vi "dI-dV(V) at various H_MFLI_MF-MD_K3636B(channelB)_measureX_PK_V4.0_withaveraging.vi"() -> ()   [LabVIEW 2016]
uses:
  <instrlib>/Zurich Instruments LabOne/Public/Data/ziTypeDemodSampleSingle.ctl
  <instrlib>/Keithley 2600 Series/Public/Configure/Source/Configure Source (Limit).vi
  <instrlib>/Keithley 2600 Series/Public/Configure/Source/Configure Source (Range).vi
  <instrlib>/Zurich Instruments LabOne/Public/Configure/ziSetValueDouble.vi
  <instrlib>/Zurich Instruments LabOne/Public/Configure/ziGetValueDemodSampleEx.vi
  <instrlib>/Zurich Instruments LabOne/Zurich Instruments LabOne.lvlib
  <instrlib>/Keithley 2600 Series/Keithley 2600 Series.lvlib
panel:
  in  "MFLI autophase":bool
  in  "MFLI autorange":bool
  in  "MFLI averaging":i32=20
  in  "Resistance used for DC (ohm)":dbl=20000000.0 format="%#_13g"
  in  "DC Current Limit (A)":dbl=0.001 format="%#_13g"
  in  "Keithley 2636B (channelB)":refnum<visa-resource-name>="GPIB0::26::INSTR"
  in  "Field ramp rate (T/min)":string="0.05"
  in  "Step 2":dbl[](array[numeric])=[0.01] min=-3000.0 max=3000.0 format="%.1e"
  in  "To 2":dbl[](array[numeric])=[0.3] min=-3000.0 max=3000.0 format="%.1e"
  in  "From 2":dbl[](array[numeric])=[0.0] min=-3000.0 max=3000.0 format="%.1e"
  in  "Magnet IP Address":string="169.254.13.196"
  in  "Magnetic field stabilization time (s)":dbl=10.0 format="%#_13g"
  out "Magnetic Field (T)":dbl=-3.778e-06 format="%#_13g"
  in  "DC Voltage averaging":dbl=20.0 format="%#_13g"
  out "Demod Sample Out 2":T1={"Timestamps (ticks)"=128778643837950, "X (Vrms)"=2.3166004932731997e-10, "Y (Vrms)"=-1.6838016027024e-10, "Osc Phase (deg)"=2.502497907836938, "Freq (Hz)"=137.91900016713043, "DIO"=0, "AuxIn0 (V)"=-1.6014270555751864, "AuxIn1 (V)"=0.0003336581285111606, "Trigger"=768}
  out "Demod Sample Out":T1={"Timestamps (ticks)"=128778342710270, "X (Vrms)"=1.6896364938522627e-05, "Y (Vrms)"=-1.248107801044493e-05, "Osc Phase (deg)"=1.3353302758544507, "Freq (Hz)"=137.91900016713043, "DIO"=0, "AuxIn0 (V)"=-1.6014270555751864, "AuxIn1 (V)"=-0.0013346325140446424, "Trigger"=0}
  out "Vset (V)":dbl=-1.5999999999999879
  in  "stop":bool
  out "Time(s)":dbl=17571.544
  in  "Delay (s)":dbl=4.0
  out "dI/dV (S)":dbl=1.3582224457345251e-05
  out "dV (V)":dbl=1.6935759280791425e-05
  out "dI (A)":dbl=2.300252839072771e-10
  in  "MFLI Address":string="DEV4496"
  out "DC Voltage (V)":dbl=0.0024181997905000007
  in  "Folder":path=path "D:/Pranava/Data/Pt-Co-Ta/25-05-2021"
  out "dI/dV vs DC Bias (V)":cluster{dbl, "Field Reading":dbl}[](graph)=[{-0.001627013885, "Field Reading"=1.6344764120468297e-05}, {-0.001619012798, "Field Reading"=1.3998765196903891e-05}, {-0.0016148306399999999, "Field Reading"=1.3700556199628512e-05}, {-0.0016116390899999999, "Field Reading"=1.3871656998400836e-05}, {-0.0016093190579999999, "Field Reading"=1.3890284519929273e-05}, {-0.0016034726325000002, "Field Reading"=1.3832673860262865e-05}, {-0.0016014351899999997, "Field Reading"=1.3751553995812428e-05}, {-0.0015951204535000004, "Field Reading"=1.3732003453418088e-05}, {-0.001597877244, "Field Reading"=1.3898216235721011e-05}, {-0.0015940734674999998, "Field Reading"=1.3997320460561689e-05}, {-0.0015882617540000001, "Field Reading"=1.3508618550371427e-05}, {-0.0015828277630000002, "Field Reading"=1.367402259462331e-05}, {-0.0015791635179999998, "Field Reading"=1.3527207584083079e-05}, {-0.0015766756889999997, "Field Reading"=1.3882099502793414e-05}, {-0.00157194422, "Field Reading"=1.3768418031370217e-05}, {-0.0015670328779999998, "Field Reading"=1.364782208277766e-05}, {-0.0015644425175, "Field Reading"=1.3804633828353077e-05}, {-0.001564032793, "Field Reading"=1.3888199858922033e-05}, {-0.001557341777, "Field Reading"=1.3614302852212391e-05}, {-0.001552385615, "Field Reading"=1.3810158703062188e-05}, {-0.0015469061994999999, "Field Reading"=1.3764713120794011e-05}, {-0.001546229423, "Field Reading"=1.369552113795401e-05}, {-0.0015404441190000001, "Field Reading"=1.3693812113712007e-05}, {-0.0015395130355, "Field Reading"=1.3781883943418925e-05}, {-0.0015314868149999999, "Field Reading"=1.3770965025421842e-05}, {-0.0015304288265, "Field Reading"=1.3798857346413868e-05}, {-0.001527220823, "Field Reading"=1.3715545304114617e-05}, {-0.0015249214555, "Field Reading"=1.3691708736082112e-05}, {-0.0015218840245, "Field Reading"=1.3708493049006325e-05}, {-0.001520791987, "Field Reading"=1.3817916720703356e-05}, {-0.0015147427645, "Field Reading"=1.3894961593511675e-05}, {-0.001517215882, "Field Reading"=1.3590033991382936e-05}, {-0.0015114531689999998, "Field Reading"=1.3756144247138902e-05}, {-0.0015093745215, "Field Reading"=1.377966465179012e-05}, {-0.001500627891, "Field Reading"=1.3951323244665344e-05}, {-0.0015025901485, "Field Reading"=1.3667118977084549e-05}, {-0.0014961112455, "Field Reading"=1.3773922587587749e-05}, {-0.001492517136, "Field Reading"=1.3885930772190326e-05}, {-0.0014830039544999998, "Field Reading"=1.401422781639763e-05}, {-0.0014816401655, "Field Reading"=1.397897771474187e-05}, {-0.00147841159, "Field Reading"=1.379012752602543e-05}, {-0.0014741321355, "Field Reading"=1.3677898377939856e-05}, {-0.0014710702515, "Field Reading"=1.3843469527200954e-05}, {-0.0014655690059999999, "Field Reading"=1.3916776180729468e-05}, {-0.0014595854975000002, "Field Reading"=1.3757666149806165e-05}, {-0.0014580961389999997, "Field Reading"=1.3700038667069656e-05}, {-0.0014554962550000002, "Field Reading"=1.3953242012805934e-05}, {-0.0014536663915, "Field Reading"=1.3900636198435842e-05}, {-0.0014442646640000002, "Field Reading"=1.3742972292234844e-05}, {-0.001445856694, "Field Reading"=1.3937226017817598e-05}, {-0.0014406852145, "Field Reading"=1.3857514292073597e-05}, {-0.0014354871654999998, "Field Reading"=1.4045929404858086e-05}, {-0.001434501668, "Field Reading"=1.4042163913670806e-05}, {-0.0014285742130000002, "Field Reading"=1.3914255657909023e-05}, {-0.001420600119, "Field Reading"=1.3960330416901324e-05}, {-0.00142239087, "Field Reading"=1.387496710959369e-05}, {-0.001420244116, "Field Reading"=1.3967109128526288e-05}, {-0.0014127562885, "Field Reading"=1.3875867237048908e-05}, {-0.001408771663, "Field Reading"=1.371589748742955e-05}, {-0.001407767006, "Field Reading"=1.3711464298673438e-05}, {-0.0014066237619999998, "Field Reading"=1.359596749779307e-05}, {-0.0013982159850000001, "Field Reading"=1.353920245984042e-05}, {-0.001394893425, "Field Reading"=1.3670386134660128e-05}, {-0.001394967168, "Field Reading"=1.3821642182251017e-05}, {-0.0013881122135, "Field Reading"=1.3729902840276138e-05}, {-0.0013830394475, "Field Reading"=1.3556381296841854e-05}, {-0.0013815175825, "Field Reading"=1.3785118649184657e-05}, {-0.0013814490670000003, "Field Reading"=1.3640417617186004e-05}, {-0.001377212742, "Field Reading"=1.3771308247335462e-05}, {-0.0013776005575, "Field Reading"=1.3917559046858347e-05}, {-0.0013736268475, "Field Reading"=1.3546940902423523e-05}, {-0.0013717613320000002, "Field Reading"=1.3689011639519566e-05}, {-0.0013626009480000002, "Field Reading"=1.3568629924474036e-05}, {-0.0013606890300000003, "Field Reading"=1.35011849360303e-05}, {-0.0013540541445, "Field Reading"=1.367825161699194e-05}, {-0.0013570977190000002, "Field Reading"=1.3519671249396716e-05}, {-0.0013493867404999998, "Field Reading"=1.3709253795395331e-05}, {-0.001344058568, "Field Reading"=1.3634845505302235e-05}, {-0.001339602049, "Field Reading"=1.3360159655150527e-05}, {-0.0013348508405000002, "Field Reading"=1.3545439977833426e-05}, {-0.0013321022040000002, "Field Reading"=1.3499265468607369e-05}, {-0.0013296686680000001, "Field Reading"=1.3712801766846765e-05}, {-0.0013238164165, "Field Reading"=1.3620193842710997e-05}, {-0.001326682167, "Field Reading"=1.3429530329586303e-05}, {-0.0013223496344999999, "Field Reading"=1.348118208734371e-05}, {-0.0013149475535, "Field Reading"=1.3473355677728207e-05}, {-0.0013093518845, "Field Reading"=1.343488469738469e-05}, {-0.0013077079579999998, "Field Reading"=1.340487335540023e-05}, {-0.001302729128, "Field Reading"=1.3271641453823996e-05}, {-0.0013011367614999998, "Field Reading"=1.3256838231012924e-05}, {-0.001296205141, "Field Reading"=1.3414108723421038e-05}, {-0.001292995518, "Field Reading"=1.3259760334792129e-05}, {-0.001286491578, "Field Reading"=1.3500648663763856e-05}, {-0.001280819065, "Field Reading"=1.3411728157299298e-05}, {-0.001275759533, "Field Reading"=1.3379940620171237e-05}, {-0.001278334064, "Field Reading"=1.3288518867407855e-05}, {-0.001277028731, "Field Reading"=1.3517866434305292e-05}, {-0.001271280125, "Field Reading"=1.3148021252298002e-05}, {-0.0012640221705, "Field Reading"=1.3278150097955834e-05}, {-0.0012593509910000002, "Field Reading"=1.314984586996218e-05}, {-0.0012547493175, "Field Reading"=1.3060872038559914e-05}, {-0.001252087101, "Field Reading"=1.3020302107075454e-05}, {-0.0012439236884999997, "Field Reading"=1.316109299519562e-05}, {-0.0012387295854999999, "Field Reading"=1.2929870136154811e-05}, {-0.0012391171569999999, "Field Reading"=1.3089890985118604e-05}, {-0.001234343349, "Field Reading"=1.3097514711203912e-05}, {-0.0012290445895, "Field Reading"=1.2921869305819281e-05}, {-0.001229663533, "Field Reading"=1.2862993431135441e-05}, {-0.001229092529, "Field Reading"=1.2984016389860433e-05}, {-0.0012203022500000002, "Field Reading"=1.2903660255895865e-05}, {-0.001218487702, "Field Reading"=1.295229292926011e-05}, {-0.0012142243634999997, "Field Reading"=1.2945524197075967e-05}, {-0.0012130919644999997, "Field Reading"=1.2975531697804405e-05}, {-0.0012090447284999997, "Field Reading"=1.2897127188873693e-05}, {-0.001205265464, "Field Reading"=1.3020848594089028e-05}, {-0.0011975085925, "Field Reading"=1.2872792012437228e-05}, {-0.001195983172, "Field Reading"=1.3123292853972002e-05}, {-0.0011921657645, "Field Reading"=1.275596330441878e-05}, {-0.001186216861, "Field Reading"=1.2815863244369823e-05}, {-0.0011855908475000001, "Field Reading"=1.2751096142754899e-05}, {-0.001180132249, "Field Reading"=1.2845234952429745e-05}, {-0.0011768545429999997, "Field Reading"=1.2712544584458588e-05}, {-0.0011693543635, "Field Reading"=1.2689530733941001e-05}, {-0.0011648539619999998, "Field Reading"=1.2813457056850323e-05}, {-0.0011591180770000001, "Field Reading"=1.2649561027374934e-05}, {-0.001160082554, "Field Reading"=1.2842648532994943e-05}, {-0.0011558191740000002, "Field Reading"=1.2853797849249115e-05}, {-0.0011519055545000001, "Field Reading"=1.2479763728298495e-05}, {-0.001151550178, "Field Reading"=1.2736050264332894e-05}, {-0.0011431843185, "Field Reading"=1.2681891931039486e-05}, {-0.0011405739945, "Field Reading"=1.2670834803913829e-05}, {-0.0011361765430000002, "Field Reading"=1.264764856181773e-05}, {-0.0011358318899999998, "Field Reading"=1.2526321018150686e-05}, {-0.001133606925, "Field Reading"=1.2416807967576818e-05}, {-0.0011259585075000002, "Field Reading"=1.2555461044117877e-05}, {-0.0011249923370000002, "Field Reading"=1.246008007785992e-05}, {-0.0011250493870000001, "Field Reading"=1.248310208986633e-05}, {-0.0011180441384999998, "Field Reading"=1.2463593264951724e-05}, {-0.0011139388929999998, "Field Reading"=1.2755848980959075e-05}, {-0.0011092396729999996, "Field Reading"=1.278223306962051e-05}, {-0.0011031808695, "Field Reading"=1.2378999975066592e-05}, {-0.001098872621, "Field Reading"=1.2355079517708083e-05}, {-0.0010941898799999997, "Field Reading"=1.273445222705829e-05}, {-0.0010883913155, "Field Reading"=1.2630177622571002e-05}, {-0.0010851332794999998, "Field Reading"=1.2410535404675337e-05}, {-0.0010825103265, "Field Reading"=1.2641276509599764e-05}, {-0.001079658241, "Field Reading"=1.2520377620495749e-05}, {-0.0010739608169999999, "Field Reading"=1.2357646860773063e-05}, {-0.0010726618789999999, "Field Reading"=1.2602802293707646e-05}, {-0.0010694978194999997, "Field Reading"=1.2494598777705452e-05}, {-0.0010631378544999999, "Field Reading"=1.2301982558271114e-05}, {-0.001057875101, "Field Reading"=1.237560383349787e-05}, {-0.0010562695905000001, "Field Reading"=1.2512748983290444e-05}, {-0.0010508747024999998, "Field Reading"=1.2333035389988188e-05}, {-0.0010451592750000001, "Field Reading"=1.2370779967336252e-05}, {-0.0010449503275, "Field Reading"=1.2683917677046795e-05}, {-0.0010374406835, "Field Reading"=1.2307116274430603e-05}, {-0.0010297802020000004, "Field Reading"=1.2470968278406303e-05}, {-0.0010274126785, "Field Reading"=1.2676998220006918e-05}, {-0.0010244289280000002, "Field Reading"=1.2684575834320789e-05}, {-0.001019885346, "Field Reading"=1.2574404115195829e-05}, {-0.0010140041260000004, "Field Reading"=1.2588632490089326e-05}, {-0.0010120979235, "Field Reading"=1.266325189583356e-05}, {-0.0010068855770000002, "Field Reading"=1.2397082577085974e-05}, {-0.0010022195958, "Field Reading"=1.2825417366117891e-05}, {-0.0009982523001999999, "Field Reading"=1.2575009416285682e-05}, {-0.0009985486988000002, "Field Reading"=1.2641165343983029e-05}, {-0.0009910957783000002, "Field Reading"=1.250657455312929e-05}, {-0.0009924337100500002, "Field Reading"=1.2727936948495928e-05}, {-0.0009877553554, "Field Reading"=1.2701889527060823e-05}, {-0.0009858346862999998, "Field Reading"=1.2789594077695873e-05}, {-0.000976561241, "Field Reading"=1.2545928182264849e-05}, {-0.0009763876650999998, "Field Reading"=1.2565889150967984e-05}, {-0.0009659327763, "Field Reading"=1.2494168705440488e-05}, {-0.0009642664521500001, "Field Reading"=1.277044835111768e-05}, {-0.0009606519217999999, "Field Reading"=1.2621458517459202e-05}, {-0.0009539253218000001, "Field Reading"=1.2541865843016244e-05}, {-0.0009544971631999999, "Field Reading"=1.2856460131262982e-05}, {-0.0009503665630499999, "Field Reading"=1.2637052604573622e-05}, {-0.0009470002221499999, "Field Reading"=1.2409391364210763e-05}, {-0.0009472342232999997, "Field Reading"=1.2812128060793574e-05}, {-0.0009404217817500001, "Field Reading"=1.2517373602241441e-05}, {-0.0009362671446500002, "Field Reading"=1.2752817377595242e-05}, {-0.0009295569483500002, "Field Reading"=1.2870775933596313e-05}, {-0.0009233142658000001, "Field Reading"=1.2940782105266904e-05}, {-0.0009272410244499998, "Field Reading"=1.2864982761510018e-05}, {-0.0009218127019000001, "Field Reading"=1.2791592310478834e-05}, {-0.0009178675715, "Field Reading"=1.2844351835678336e-05}, {-0.00091000123255, "Field Reading"=1.2905873397991618e-05}, {-0.00090152457665, "Field Reading"=1.2611711679497694e-05}, {-0.0009011194442499999, "Field Reading"=1.2583618150960818e-05}, {-0.0008935033273, "Field Reading"=1.2508511442445113e-05}, {-0.0008944143545999998, "Field Reading"=1.2746451142201546e-05}, {-0.0008970966182500001, "Field Reading"=1.272818905705432e-05}, {-0.0008852390063500002, "Field Reading"=1.283242639342165e-05}, {-0.00088406414315, "Field Reading"=1.2589059858355413e-05}, {-0.0008745983877499998, "Field Reading"=1.2872289514291092e-05}, {-0.0008714598008000001, "Field Reading"=1.2669941304728081e-05}, {-0.0008709556687999999, "Field Reading"=1.2539001686833629e-05}, {-0.000868388288, "Field Reading"=1.2521844511669537e-05}, {-0.0008664498490499999, "Field Reading"=1.2805259841152486e-05}, {-0.0008643681782500001, "Field Reading"=1.2529815581555094e-05}, {-0.0008561518372, "Field Reading"=1.2686854791708634e-05}, {-0.0008526448225, "Field Reading"=1.243150088195482e-05}, {-0.00084623768195, "Field Reading"=1.2385322813511503e-05}, {-0.00084599694325, "Field Reading"=1.2205326451618826e-05}, {-0.0008395531274499998, "Field Reading"=1.2440860523822803e-05}, {-0.0008281302789499999, "Field Reading"=1.2439894342151496e-05}, {-0.0008248335999500001, "Field Reading"=1.2424045335858269e-05}, {-0.0008203613541, "Field Reading"=1.2144269058622703e-05}, {-0.0008234964726500001, "Field Reading"=1.2233044327647624e-05}, {-0.0008169651179000001, "Field Reading"=1.2109231360596383e-05}, {-0.0008122484677, "Field Reading"=1.2120033499666712e-05}, {-0.0008110532533000001, "Field Reading"=1.1857849084584533e-05}, {-0.0008057847579000001, "Field Reading"=1.1766175681406275e-05}, {-0.0007990924092, "Field Reading"=1.1772956497108558e-05}, {-0.0007923443377, "Field Reading"=1.182771265435658e-05}, {-0.00079106090435, "Field Reading"=1.1580989325589795e-05}, {-0.00078530423725, "Field Reading"=1.1446076295068069e-05}, {-0.0007878125519999999, "Field Reading"=1.1359632652403681e-05}, {-0.0007791636374, "Field Reading"=1.1371644502308576e-05}, {-0.0007729273194, "Field Reading"=1.1121496876365996e-05}, {-0.0007658445544499999, "Field Reading"=1.0951708685534248e-05}, {-0.0007586431640999999, "Field Reading"=1.1076989094457801e-05}, {-0.00075945477685, "Field Reading"=1.081289845032397e-05}, {-0.0007581331682, "Field Reading"=1.0791931490640528e-05}, {-0.0007532736652, "Field Reading"=1.0495729701910961e-05}, {-0.0007462233425000001, "Field Reading"=1.0386855215343259e-05}, {-0.00074202178005, "Field Reading"=1.0263689725134089e-05}, {-0.0007400187412, "Field Reading"=1.0416055155919835e-05}, {-0.00073782228595, "Field Reading"=9.951225216108973e-06}, {-0.0007311943481000001, "Field Reading"=9.903494680663152e-06}, {-0.0007205318164000001, "Field Reading"=9.963488153334e-06}, {-0.0007154980816999999, "Field Reading"=9.810708954565177e-06}, {-0.0007125741843500001, "Field Reading"=9.706610299848867e-06}, {-0.00070746760055, "Field Reading"=9.441744804879048e-06}, {-0.0007013541408499999, "Field Reading"=8.84923943591659e-06}, {-0.0006984238498, "Field Reading"=8.875472436899315e-06}, {-0.0006907229907000001, "Field Reading"=8.699519253679955e-06}, {-0.0006808327704, "Field Reading"=8.833569750798664e-06}, {-0.0006847265971, "Field Reading"=8.543177441919965e-06}, {-0.00067869460815, "Field Reading"=8.315767516705057e-06}, {-0.00067265827835, "Field Reading"=8.062355332923912e-06}, {-0.0006669619085, "Field Reading"=7.901811353466826e-06}, {-0.000658885147, "Field Reading"=7.879441057954235e-06}, {-0.0006545641374, "Field Reading"=8.09911974210054e-06}, {-0.0006444034975000001, "Field Reading"=7.854339480468222e-06}, {-0.0006348567222, "Field Reading"=7.866445287086442e-06}, {-0.00062975573455, "Field Reading"=7.546732494702164e-06}, {-0.0006282009054000001, "Field Reading"=7.671978484770857e-06}, {-0.000627307381, "Field Reading"=7.828811660063022e-06}, {-0.0006273580275000001, "Field Reading"=7.700197580007255e-06}, {-0.0006248321563500001, "Field Reading"=7.653399442051351e-06}, {-0.0006275858704, "Field Reading"=7.5627527424580506e-06}, {-0.0006309341548500001, "Field Reading"=7.583242130138117e-06}, {-0.0006285488479, "Field Reading"=7.641930571883218e-06}, {-0.00062230268925, "Field Reading"=7.87495509025875e-06}, {-0.00062258856105, "Field Reading"=7.720759005146535e-06}, {-0.0006204475316, "Field Reading"=7.662467273504187e-06}, {-0.0006225688469, "Field Reading"=7.511758391442685e-06}, {-0.00061953980585, "Field Reading"=7.103640992096702e-06}, {-0.0006164522959499999, "Field Reading"=7.431365971587332e-06}, {-0.00061573231445, "Field Reading"=7.150212317104851e-06}, {-0.0006141728360499999, "Field Reading"=7.671752339815932e-06}, {-0.00061563870065, "Field Reading"=7.414022842881697e-06}, {-0.00061160168935, "Field Reading"=7.371259342297242e-06}, {-0.0006079315858000001, "Field Reading"=7.356083800783647e-06}, {-0.0006029981042999999, "Field Reading"=7.247074149056172e-06}, {-0.00060178471345, "Field Reading"=6.829184558139492e-06}, {-0.00060771892745, "Field Reading"=7.397468909021597e-06}, {-0.00060001967735, "Field Reading"=7.497676238555896e-06}, {-0.00059898530125, "Field Reading"=7.332830670951728e-06}, {-0.0005985643774000001, "Field Reading"=7.196148037919119e-06}, {-0.0005958760605500001, "Field Reading"=7.233638643853758e-06}, {-0.0005940818876499999, "Field Reading"=7.296678288385437e-06}, {-0.0005935160713, "Field Reading"=7.13108557239412e-06}, {-0.00059269686995, "Field Reading"=7.305544686867979e-06}, {-0.0005930560289, "Field Reading"=7.193315300528358e-06}, {-0.0005861046275500001, "Field Reading"=7.0448479767246175e-06}, {-0.0005911481135000001, "Field Reading"=7.058262997625237e-06}, {-0.0005852575183000001, "Field Reading"=7.055918386433692e-06}, {-0.0005848876788, "Field Reading"=6.952050720888041e-06}, {-0.0005792974193499999, "Field Reading"=7.516006493893935e-06}, {-0.0005802494432999999, "Field Reading"=7.123367497704594e-06}, {-0.0005756203558500001, "Field Reading"=6.813354964978354e-06}, {-0.0005771658074, "Field Reading"=6.88809537733843e-06}, {-0.0005775387188, "Field Reading"=7.008728084495102e-06}, {-0.0005697983366, "Field Reading"=7.162692017777295e-06}, {-0.0005680916780000001, "Field Reading"=7.020017262273062e-06}, {-0.0005703411884, "Field Reading"=6.852967798722027e-06}, {-0.0005682610610500002, "Field Reading"=6.983133991727153e-06}, {-0.00057034519845, "Field Reading"=6.847443158606952e-06}, {-0.0005707841498, "Field Reading"=6.829456288676907e-06}, {-0.0005700667513999999, "Field Reading"=6.654403241523341e-06}, {-0.0005681158123999999, "Field Reading"=6.838568121688521e-06}, {-0.0005673089191500001, "Field Reading"=6.7693227845362525e-06}, {-0.0005655302658500001, "Field Reading"=6.778950995459109e-06}, {-0.0005611021443000001, "Field Reading"=6.729476968313962e-06}, {-0.0005616331016, "Field Reading"=6.604772436238808e-06}, {-0.00055700269345, "Field Reading"=6.844096294949602e-06}, {-0.0005576420179999999, "Field Reading"=6.770244836003932e-06}, {-0.0005541664579999999, "Field Reading"=6.886890283890427e-06}, {-0.0005594620287, "Field Reading"=6.738182044625657e-06}, {-0.0005598049227999999, "Field Reading"=6.900226770683148e-06}, {-0.0005581776121000001, "Field Reading"=6.78861799384101e-06}, {-0.0005478216878000001, "Field Reading"=6.666731831705923e-06}, {-0.0005480996190999999, "Field Reading"=6.647047344041987e-06}, {-0.0005490282680999999, "Field Reading"=6.702860084656656e-06}, {-0.000546962741, "Field Reading"=6.728239971040004e-06}, {-0.0005440506501999999, "Field Reading"=6.82012559268769e-06}, {-0.0005421423742, "Field Reading"=6.675778433559204e-06}, {-0.00054192168355, "Field Reading"=6.634353954560173e-06}, {-0.00053588011205, "Field Reading"=6.621880685945069e-06}, {-0.0005359785913499999, "Field Reading"=6.772030493885964e-06}, {-0.0005335594295, "Field Reading"=6.607228689308569e-06}, {-0.0005340741782, "Field Reading"=6.686141510241689e-06}, {-0.0005318644251999999, "Field Reading"=6.795320173237086e-06}, {-0.0005296052244500001, "Field Reading"=6.714946694612993e-06}, {-0.00052749707175, "Field Reading"=6.608628089694611e-06}, {-0.0005271789118, "Field Reading"=6.599566789457984e-06}, {-0.0005274487263000001, "Field Reading"=6.657735603416196e-06}, {-0.0005318625882500001, "Field Reading"=6.690153435918709e-06}, {-0.00052698555925, "Field Reading"=6.596279550132335e-06}, {-0.0005238467298, "Field Reading"=6.676241094033141e-06}, {-0.00051937956735, "Field Reading"=6.850864079430735e-06}, {-0.0005161447851, "Field Reading"=6.705803255050683e-06}, {-0.00051423159645, "Field Reading"=6.6601072939865385e-06}, {-0.0005178000224500001, "Field Reading"=6.748773246992164e-06}, {-0.0005161715310999999, "Field Reading"=6.6876638275565215e-06}, {-0.00051069515145, "Field Reading"=6.784590387488596e-06}, {-0.00051336694125, "Field Reading"=6.786092556581579e-06}, {-0.0005113064408, "Field Reading"=6.8065150289387e-06}, {-0.00051379582785, "Field Reading"=6.561251556608021e-06}, {-0.00051116757795, "Field Reading"=6.845233966083136e-06}, {-0.0005147050454000001, "Field Reading"=6.7421900282745465e-06}, {-0.0005159687170999999, "Field Reading"=6.798635998422379e-06}, {-0.0005105977054, "Field Reading"=6.7763307855727e-06}, {-0.0005119236264, "Field Reading"=6.736451450388616e-06}, {-0.00050839933305, "Field Reading"=6.7678042709707144e-06}, {-0.00050455272905, "Field Reading"=6.7947027101116485e-06}, {-0.000500762708, "Field Reading"=6.846962905547986e-06}, {-0.0004986285368, "Field Reading"=6.667799780583689e-06}, {-0.00049574743765, "Field Reading"=6.6585759435283586e-06}, {-0.0005001396443499999, "Field Reading"=6.781045968686815e-06}, {-0.0004966048467500001, "Field Reading"=6.856656492598681e-06}, {-0.0004972405634499999, "Field Reading"=6.781527696078811e-06}, {-0.0004923580213499999, "Field Reading"=6.776511137432092e-06}, {-0.0004917653571499999, "Field Reading"=6.775142991697667e-06}, {-0.0004922742916, "Field Reading"=6.7844200528519425e-06}, {-0.00048800341875, "Field Reading"=6.723039782942214e-06}, {-0.0004873660292, "Field Reading"=6.94129650875661e-06}, {-0.0004846360536000001, "Field Reading"=6.941546203008168e-06}, {-0.00048486909605, "Field Reading"=6.940101046988942e-06}, {-0.00048368177494999997, "Field Reading"=6.976172313698844e-06}, {-0.0004824013804499999, "Field Reading"=6.924376262738316e-06}, {-0.00048069004349999997, "Field Reading"=6.887033627621488e-06}, {-0.00048085519405, "Field Reading"=7.001307626185981e-06}, {-0.0004712860013499999, "Field Reading"=7.111149643385221e-06}, {-0.00047676863494999994, "Field Reading"=6.9842676042005655e-06}, {-0.00047288857814999996, "Field Reading"=6.9116078038669506e-06}, {-0.0004751365217, "Field Reading"=7.066244363459512e-06}, {-0.0004684349262999999, "Field Reading"=7.046542407700389e-06}, {-0.00046194838535000007, "Field Reading"=7.121085938299403e-06}, {-0.00045883218019999994, "Field Reading"=7.032415692863838e-06}, {-0.00045618192274999995, "Field Reading"=7.187905091896904e-06}, {-0.0004623354443000001, "Field Reading"=7.059877345434046e-06}, {-0.0004622446008999999, "Field Reading"=7.077582321279902e-06}, {-0.0004612278872, "Field Reading"=7.074631934941284e-06}, {-0.00046082623119999996, "Field Reading"=7.078778675890706e-06}, {-0.00045794411325, "Field Reading"=7.269043360665607e-06}, {-0.00046034955325, "Field Reading"=7.357617186009114e-06}, {-0.00045435257584999994, "Field Reading"=7.47732098362762e-06}, {-0.00045655454895, "Field Reading"=7.2383224064065385e-06}, {-0.00045224840289999997, "Field Reading"=7.300225716648718e-06}, {-0.00045578147750000004, "Field Reading"=7.212816135541476e-06}, {-0.00044912568584999993, "Field Reading"=7.561046173353483e-06}, {-0.00045090267219999997, "Field Reading"=7.2369275471574086e-06}, {-0.00045528761669999995, "Field Reading"=7.281461940825961e-06}, {-0.00045202417114999997, "Field Reading"=7.401916789101538e-06}, {-0.00045722160114999996, "Field Reading"=7.331725694458896e-06}, {-0.00044884362665, "Field Reading"=7.4010499213862446e-06}, {-0.00045165789110000005, "Field Reading"=7.4474942962048565e-06}, {-0.00044335969930000006, "Field Reading"=7.327169341246536e-06}, {-0.00043860972815, "Field Reading"=7.76948941998839e-06}, {-0.00043716359120000005, "Field Reading"=7.861722974292615e-06}, {-0.00043949798629999996, "Field Reading"=7.748604797824077e-06}, {-0.0004363722307999999, "Field Reading"=7.3963780284318356e-06}, {-0.00043668675275, "Field Reading"=7.4480762613215185e-06}, {-0.00043649516409999993, "Field Reading"=7.745117578937036e-06}, {-0.00043287416999999995, "Field Reading"=7.654214299900013e-06}, {-0.00043082809590000003, "Field Reading"=7.700349424629718e-06}, {-0.00043158282435000006, "Field Reading"=7.664556933051392e-06}, {-0.00042314650950000003, "Field Reading"=7.902578231021132e-06}, {-0.00041940969135, "Field Reading"=7.953587703961766e-06}, {-0.00042515681325000005, "Field Reading"=7.906381284995515e-06}, {-0.00043026784555000004, "Field Reading"=7.615834073699331e-06}, {-0.00042418069265, "Field Reading"=7.69394125684261e-06}, {-0.00042384930384999997, "Field Reading"=7.846277331020805e-06}, {-0.00042096776065, "Field Reading"=7.777029297975918e-06}, {-0.00042474697220000007, "Field Reading"=7.763165846419434e-06}, {-0.0004184529625, "Field Reading"=7.725457879461285e-06}, {-0.0004194809252499999, "Field Reading"=7.71869473167376e-06}, {-0.00041409541680000007, "Field Reading"=8.019122526464664e-06}, {-0.00041207677845, "Field Reading"=7.837579528286606e-06}, {-0.00040358748015, "Field Reading"=8.00603863466651e-06}, {-0.00041114110174999993, "Field Reading"=8.015057496183957e-06}, {-0.00040982928405, "Field Reading"=7.925350821028377e-06}, {-0.00040613316139999996, "Field Reading"=7.952069024799839e-06}, {-0.0004093220320500001, "Field Reading"=8.043703812652882e-06}, {-0.00040936323505, "Field Reading"=8.031835199165312e-06}, {-0.0004046772355999999, "Field Reading"=8.118712247107399e-06}, {-0.000405243221, "Field Reading"=8.067324993982773e-06}, {-0.00040396662685, "Field Reading"=8.080977859265871e-06}, {-0.0004023183884499999, "Field Reading"=8.186888491188982e-06}, {-0.00040208404475, "Field Reading"=8.193631222969814e-06}, {-0.0004021506078, "Field Reading"=8.088140289322153e-06}, {-0.00040174244749999996, "Field Reading"=8.022202192050063e-06}, {-0.0004038975091, "Field Reading"=8.151544548150494e-06}, {-0.00040206298985000005, "Field Reading"=8.264812942390961e-06}, {-0.00039910128009999996, "Field Reading"=8.234019525393471e-06}, {-0.0003951889136999999, "Field Reading"=8.230585505412914e-06}, {-0.00039219545584999997, "Field Reading"=8.502456135355299e-06}, {-0.000389174097, "Field Reading"=8.225247031737236e-06}, {-0.00039048983784999993, "Field Reading"=8.143176371279353e-06}, {-0.00039093352474999996, "Field Reading"=8.366502003890328e-06}, {-0.00038847995755000007, "Field Reading"=8.289844234130168e-06}, {-0.00038754884195, "Field Reading"=8.334928238438704e-06}, {-0.00037909900170000004, "Field Reading"=8.26737216855091e-06}, {-0.0003819473534, "Field Reading"=8.323216408197008e-06}, {-0.00038179316995, "Field Reading"=8.524506685045283e-06}, {-0.00037617638075, "Field Reading"=8.627150615499936e-06}, {-0.00037517814555000005, "Field Reading"=8.455366535513593e-06}, {-0.00038091039375, "Field Reading"=8.444981924747903e-06}, {-0.0003768191683, "Field Reading"=8.571976472860457e-06}, {-0.00037777723424999997, "Field Reading"=8.614701976109057e-06}, {-0.00037084848195, "Field Reading"=8.632036936843344e-06}, {-0.00037184744695000003, "Field Reading"=8.660504417506411e-06}, {-0.00037758249055, "Field Reading"=8.383352428703526e-06}, {-0.0003668550456, "Field Reading"=8.84018563341687e-06}, {-0.00036771338025, "Field Reading"=8.789321659582276e-06}, {-0.0003682380523, "Field Reading"=8.68898613774474e-06}, {-0.0003642330111, "Field Reading"=8.897586723885342e-06}, {-0.0003643684847, "Field Reading"=8.692551526596216e-06}, {-0.00036233132264999995, "Field Reading"=8.791396503412202e-06}, {-0.0003595674064, "Field Reading"=8.434820283433495e-06}, {-0.0003629669301, "Field Reading"=8.828156000823983e-06}, {-0.00036074512280000003, "Field Reading"=8.640647411171717e-06}, {-0.00035823619875, "Field Reading"=8.524945476083626e-06}, {-0.00035970884175, "Field Reading"=8.679453874203654e-06}, {-0.0003600435608, "Field Reading"=8.578955035194646e-06}, {-0.00036079289785, "Field Reading"=8.543275386069665e-06}, {-0.00036176898445000003, "Field Reading"=8.558724513556256e-06}, {-0.00035501890774999997, "Field Reading"=8.473271606533991e-06}, {-0.00034792710570000007, "Field Reading"=8.55386374973395e-06}, {-0.00035021135765, "Field Reading"=8.688751461279344e-06}, {-0.0003470909623, "Field Reading"=8.62421355151374e-06}, {-0.00034682714435, "Field Reading"=8.619585597616744e-06}, {-0.0003471232492, "Field Reading"=8.593008729168896e-06}, {-0.00034590277215, "Field Reading"=8.499236176350022e-06}, {-0.0003469728986, "Field Reading"=8.691761989372852e-06}, {-0.00034243741759999995, "Field Reading"=8.871103679662337e-06}, {-0.00034415307555, "Field Reading"=8.784065447539836e-06}, {-0.00033743379805, "Field Reading"=8.67532351470984e-06}, {-0.0003397425146, "Field Reading"=8.821494535463515e-06}, {-0.00033510807840000006, "Field Reading"=8.838480439816481e-06}, {-0.00033382716565, "Field Reading"=8.92855848090016e-06}, {-0.0003339950628, "Field Reading"=8.88729296390918e-06}, {-0.0003334059782, "Field Reading"=8.83164918997357e-06}, {-0.00033155857365000003, "Field Reading"=8.829405592709888e-06}, {-0.00032746315874999997, "Field Reading"=8.670334250992068e-06}, {-0.00032760911899999993, "Field Reading"=8.873934981538838e-06}, {-0.0003272559962, "Field Reading"=8.799122372370097e-06}, {-0.00032592742905, "Field Reading"=8.952786372090711e-06}, {-0.0003250078179, "Field Reading"=8.953890868107352e-06}, {-0.00032466045995, "Field Reading"=8.990574071143114e-06}, {-0.000323617791, "Field Reading"=9.05635006891137e-06}, {-0.00032814111355, "Field Reading"=9.100067947409944e-06}, {-0.00032892071990000003, "Field Reading"=9.15642797143987e-06}, {-0.00033340848845, "Field Reading"=9.020849005857293e-06}, {-0.00032571641045000003, "Field Reading"=8.911546051812933e-06}, {-0.0003245559, "Field Reading"=8.917299329475768e-06}, {-0.00032650817060000004, "Field Reading"=9.03593150590173e-06}, {-0.0003234421954, "Field Reading"=9.019796087493757e-06}, {-0.0003222660377, "Field Reading"=8.893912880405623e-06}, {-0.00032268750974999996, "Field Reading"=9.032635468383858e-06}, {-0.00031982932500000005, "Field Reading"=8.847120731839458e-06}, {-0.0003157644429, "Field Reading"=8.963837205500058e-06}, {-0.00031041493329999996, "Field Reading"=8.839870344907743e-06}, {-0.00031334152405000003, "Field Reading"=8.915115430210383e-06}, {-0.00031667701995, "Field Reading"=9.093612632417336e-06}, {-0.00031143297680000004, "Field Reading"=8.868193320913902e-06}, {-0.00031314769725, "Field Reading"=9.146106672574902e-06}, {-0.00031165952870000006, "Field Reading"=8.82850291384161e-06}, {-0.00031124046049999996, "Field Reading"=8.749289510476604e-06}, {-0.00031014232209999995, "Field Reading"=8.820799979602393e-06}, {-0.00030976639910000007, "Field Reading"=8.792319457275106e-06}, {-0.0003091124092, "Field Reading"=8.82219565731724e-06}, {-0.000310122264, "Field Reading"=8.863450850650407e-06}, {-0.00030852876415000003, "Field Reading"=8.909221233399072e-06}, {-0.0003033401619, "Field Reading"=8.99688863421339e-06}, {-0.00030591625510000003, "Field Reading"=9.055191299232483e-06}, {-0.00030644126345, "Field Reading"=9.049112494892605e-06}, {-0.00030798667575, "Field Reading"=9.194989372010707e-06}, {-0.00030469915835, "Field Reading"=9.03267939316628e-06}, {-0.0002997061362, "Field Reading"=8.990980618815831e-06}, {-0.00029408226340000003, "Field Reading"=9.271657813541663e-06}, {-0.0002953830809, "Field Reading"=9.035342641697986e-06}, {-0.0002961272932, "Field Reading"=9.081153456956533e-06}, {-0.00029613048810000006, "Field Reading"=9.25126144436129e-06}, {-0.00029184004024999997, "Field Reading"=9.027036430480194e-06}, {-0.00029265844195000004, "Field Reading"=9.05428106017539e-06}, {-0.0002911163815, "Field Reading"=9.04373114880761e-06}, {-0.00029177830439999997, "Field Reading"=9.124224919516723e-06}, {-0.0002911989461, "Field Reading"=9.193258925044438e-06}, {-0.00028964856825, "Field Reading"=8.866762237523616e-06}, {-0.00029041938575, "Field Reading"=9.123848398759746e-06}, {-0.0002898379276, "Field Reading"=8.97118056115802e-06}, {-0.00028102725025, "Field Reading"=9.034789090026712e-06}, {-0.0002800448348, "Field Reading"=9.228187575031324e-06}, {-0.00028271463859999996, "Field Reading"=8.947807775789836e-06}, {-0.0002765786642, "Field Reading"=8.870712033484872e-06}, {-0.00027779262810000003, "Field Reading"=9.215953773914696e-06}, {-0.00028165788035, "Field Reading"=9.015900714169495e-06}, {-0.00027355756150000004, "Field Reading"=9.144430842510015e-06}, {-0.00027508150065, "Field Reading"=9.01447442062213e-06}, {-0.00027191872230000004, "Field Reading"=9.06431457285431e-06}, {-0.00027055031509999996, "Field Reading"=9.159376187412775e-06}, {-0.00026777442124999997, "Field Reading"=9.07339804527216e-06}, {-0.0002669960845, "Field Reading"=9.29592991166279e-06}, {-0.000267251843, "Field Reading"=8.98114047292202e-06}, {-0.00027045758325, "Field Reading"=9.042265476130758e-06}, {-0.00026276858735, "Field Reading"=9.056772901394442e-06}, {-0.00026654290455, "Field Reading"=9.149290903417821e-06}, {-0.00026502461985, "Field Reading"=9.012181178357452e-06}, {-0.00026557635165000003, "Field Reading"=9.108558968843962e-06}, {-0.00026223833569999995, "Field Reading"=9.040176749172146e-06}, {-0.0002661240439, "Field Reading"=9.020088117418512e-06}, {-0.00026766757909999997, "Field Reading"=9.080426891386348e-06}, {-0.000266396563, "Field Reading"=9.031973082450008e-06}, {-0.00026439926824999997, "Field Reading"=8.956605881875194e-06}, {-0.00026797944415, "Field Reading"=9.201423000132504e-06}, {-0.0002702014217, "Field Reading"=8.917061486742443e-06}, {-0.0002609158665, "Field Reading"=9.030627891163945e-06}, {-0.00025724840665, "Field Reading"=9.009870499561136e-06}, {-0.000257418023, "Field Reading"=8.778911029407525e-06}, {-0.00025517508800000004, "Field Reading"=8.892359851171787e-06}, {-0.0002513883628, "Field Reading"=8.766524313580181e-06}, {-0.00025264469965, "Field Reading"=8.407790562270027e-06}, {-0.00024839618149999994, "Field Reading"=8.718881752961406e-06}, {-0.0002457214328, "Field Reading"=8.60501291112288e-06}, {-0.00024915830085, "Field Reading"=8.741844197163829e-06}, {-0.00024499681184999997, "Field Reading"=8.44053715698851e-06}, {-0.00024477083955, "Field Reading"=8.348061004143003e-06}, {-0.00024391360219999997, "Field Reading"=8.108203951354226e-06}, {-0.00023782899894999996, "Field Reading"=8.564109351673786e-06}, {-0.00023834561559999998, "Field Reading"=8.240452440421642e-06}, {-0.00023943449594999994, "Field Reading"=8.199758339956901e-06}, {-0.00023569573974999998, "Field Reading"=7.948092833297015e-06}, {-0.0002317831752, "Field Reading"=8.043005466410338e-06}, {-0.00023345895625, "Field Reading"=8.060827210758492e-06}, {-0.00022928289659999998, "Field Reading"=7.817576231410943e-06}, {-0.00023198827479999998, "Field Reading"=7.508116843095721e-06}, {-0.00022883142975, "Field Reading"=7.36299313797122e-06}, {-0.00023008409575000005, "Field Reading"=7.540256848181872e-06}, {-0.00023239795425, "Field Reading"=7.333547283014965e-06}, {-0.00022471832489999997, "Field Reading"=7.342361601842568e-06}, {-0.00022184785754999998, "Field Reading"=7.356738690024371e-06}, {-0.00021947628525000002, "Field Reading"=7.139122010993333e-06}, {-0.00022166177774999993, "Field Reading"=7.204442620661651e-06}, {-0.00022259999559999999, "Field Reading"=7.052116709632984e-06}, {-0.0002241723121, "Field Reading"=6.982320086455824e-06}, {-0.00022044311725, "Field Reading"=6.6596879331128435e-06}, {-0.00022035598979999998, "Field Reading"=6.672409656146351e-06}, {-0.00021752159780000002, "Field Reading"=6.366832717338548e-06}, {-0.00021309576889999996, "Field Reading"=6.498829496155945e-06}, {-0.00021247514125, "Field Reading"=5.865702064733832e-06}, {-0.00021232946794999996, "Field Reading"=6.4349104550651355e-06}, {-0.00021011820484999997, "Field Reading"=6.13877191239392e-06}, {-0.00020085010665, "Field Reading"=5.904938849316602e-06}, {-0.0001991150775, "Field Reading"=5.918468364819009e-06}, {-0.00020149020544999997, "Field Reading"=5.699428471207801e-06}, {-0.00019445236944999999, "Field Reading"=5.469918295012293e-06}, {-0.00019236723165000003, "Field Reading"=5.357888879109233e-06}, {-0.00019501486445, "Field Reading"=5.189494529586777e-06}, {-0.00019323037, "Field Reading"=5.165355949893016e-06}, {-0.00018999132029999996, "Field Reading"=5.099722413214743e-06}, {-0.0001871983897, "Field Reading"=4.789929337218777e-06}, {-0.0001814051314, "Field Reading"=4.745562713297912e-06}, {-0.0001817132206, "Field Reading"=4.755517020257776e-06}, {-0.00017614730289999998, "Field Reading"=4.4244047825698195e-06}, {-0.0001727961178, "Field Reading"=3.775535144565354e-06}, {-0.0001675465376, "Field Reading"=3.802833020017866e-06}, {-0.00016431081085000002, "Field Reading"=3.91534135095458e-06}, {-0.00016157046925000004, "Field Reading"=3.5689096259221676e-06}, {-0.00016186570395, "Field Reading"=3.4715996507094622e-06}, {-0.0001607496506, "Field Reading"=3.0760437904143843e-06}, {-0.0001559256583, "Field Reading"=3.113241416545971e-06}, {-0.0001493813568, "Field Reading"=2.381228891269803e-06}, {-0.00014617880120000002, "Field Reading"=2.5898829639028055e-06}, {-0.00013571092619999998, "Field Reading"=2.337163199353694e-06}, {-0.0001329277441, "Field Reading"=2.102275965323168e-06}, {-0.0001276660733, "Field Reading"=1.7258861221078746e-06}, {-0.00011513586564999999, "Field Reading"=7.708325123652217e-07}, {-0.00010928030404999999, "Field Reading"=6.565999169577642e-07}, {-0.00010634935415000002, "Field Reading"=8.840410668664973e-07}, {-9.1024927605e-05, "Field Reading"=1.0561729184571782e-06}, {-7.119992078e-05, "Field Reading"=4.917485464759457e-07}, {-4.630999332e-05, "Field Reading"=1.385791806862855e-06}, {-4.336288705499999e-05, "Field Reading"=2.1091111306145146e-06}, {-1.4933824200500002e-05, "Field Reading"=8.723003871362913e-07}, {3.6717779650000004e-05, "Field Reading"=1.6368989353437607e-06}, {0.00019383155189999998, "Field Reading"=-1.8886276672685527e-06}, {0.0004699088057499999, "Field Reading"=7.96588441715774e-06}, {0.00066616175055, "Field Reading"=4.858965967134313e-06}, {0.0007283011614500001, "Field Reading"=-2.3556570436082966e-06}, {0.0007667300222500001, "Field Reading"=2.8288599048753896e-07}, {0.0007948254045999999, "Field Reading"=-2.949723663575285e-07}, {0.0008104692173499999, "Field Reading"=5.639919979613267e-07}, {0.0008243944047499998, "Field Reading"=1.5060937833102661e-06}, {0.0008335256873000001, "Field Reading"=1.5202690389830317e-06}, {0.0008401749466499999, "Field Reading"=1.667594323468954e-06}, {0.0008510836303000001, "Field Reading"=2.291184811840549e-06}, {0.0008515144470499999, "Field Reading"=2.470445627578318e-06}, {0.0008557425238000001, "Field Reading"=2.5512381153749575e-06}, {0.0008620111361999999, "Field Reading"=2.8040376525571e-06}, {0.0008683584158500001, "Field Reading"=3.066492545352347e-06}, {0.00087070561385, "Field Reading"=3.013416161615144e-06}, {0.00087415480725, "Field Reading"=3.512248063601155e-06}, {0.00087965760205, "Field Reading"=3.3515251015754872e-06}, {0.0008892821834500001, "Field Reading"=3.940075543844415e-06}, {0.0008882803068, "Field Reading"=4.025829079043125e-06}, {0.0008905884466, "Field Reading"=4.169570427991464e-06}, {0.00089832201945, "Field Reading"=4.108901254385864e-06}, {0.00089570786195, "Field Reading"=4.332727720840049e-06}, {0.0008970410157, "Field Reading"=4.617394689880223e-06}, {0.0009029081329499998, "Field Reading"=4.531297565617883e-06}, {0.0009078684874999998, "Field Reading"=4.541163234527896e-06}, {0.0009087108432500001, "Field Reading"=4.753827059478838e-06}, {0.0009138606843, "Field Reading"=4.752030384941524e-06}, {0.0009136408963, "Field Reading"=5.084456137724315e-06}, {0.0009169280012999998, "Field Reading"=4.875750375119563e-06}, {0.0009148154532999999, "Field Reading"=5.288686009085579e-06}, {0.0009229626562000002, "Field Reading"=5.528282291054844e-06}, {0.0009224969198999998, "Field Reading"=5.403429054237901e-06}, {0.0009294995096, "Field Reading"=5.600442328855693e-06}, {0.0009329872647500001, "Field Reading"=5.977000327232052e-06}, {0.0009320626636500002, "Field Reading"=5.76338851364554e-06}, {0.0009326099898, "Field Reading"=5.9772531015317245e-06}, {0.0009283187989999999, "Field Reading"=6.099705496056289e-06}, {0.0009404891343999999, "Field Reading"=6.069514759144942e-06}, {0.0009381479408499998, "Field Reading"=6.085266744734543e-06}, {0.0009355966974999999, "Field Reading"=6.348468923964169e-06}, {0.0009434450693499997, "Field Reading"=6.565683044019764e-06}, {0.0009432796419499999, "Field Reading"=6.637280097664824e-06}, {0.0009476389778499999, "Field Reading"=6.557470301263791e-06}, {0.0009471127507500001, "Field Reading"=6.6092743726615905e-06}, {0.0009496353743000001, "Field Reading"=6.556454921693735e-06}, {0.00094919603385, "Field Reading"=6.809181861550528e-06}, {0.0009521936217500001, "Field Reading"=6.73304206497506e-06}, {0.0009553290774499997, "Field Reading"=6.881675057596484e-06}, {0.0009547487560499999, "Field Reading"=7.073513338410298e-06}, {0.00095200275215, "Field Reading"=6.979017724679696e-06}, {0.00095860302185, "Field Reading"=7.114347340786548e-06}, {0.0009574814200500001, "Field Reading"=7.059950257896409e-06}, {0.0009556604293999999, "Field Reading"=7.0069926047761455e-06}, {0.0009603671565, "Field Reading"=7.1216029310021365e-06}, {0.000959158901, "Field Reading"=7.208152985200411e-06}, {0.0009607005388499998, "Field Reading"=7.2345421959970465e-06}, {0.0009620968772500002, "Field Reading"=7.2633043081619785e-06}, {0.0009682948202499999, "Field Reading"=7.187028478146326e-06}, {0.0009764365610500002, "Field Reading"=7.19980779755237e-06}, {0.0009871085554, "Field Reading"=7.091786424790844e-06}, {0.0009919618775, "Field Reading"=6.967883463577174e-06}, {0.0009953602116999998, "Field Reading"=6.852370153399717e-06}, {0.0010046395725, "Field Reading"=6.556044860027323e-06}, {0.0010143182605, "Field Reading"=6.388655460557607e-06}, {0.0010219913335, "Field Reading"=6.092444136434981e-06}, {0.001029279662, "Field Reading"=6.030891880101363e-06}, {0.0010371966755000001, "Field Reading"=6.048587685539682e-06}, {0.0010457810540000002, "Field Reading"=5.706885861800173e-06}, {0.001055344696, "Field Reading"=5.29670826507959e-06}, {0.0010615905040000002, "Field Reading"=5.195167824355402e-06}, {0.001076000154, "Field Reading"=4.987792116618284e-06}, {0.001084259478, "Field Reading"=4.827885633076771e-06}, {0.0010958441859999998, "Field Reading"=4.60457191390599e-06}, {0.0011081189035, "Field Reading"=4.587990789399626e-06}, {0.0011186176345, "Field Reading"=4.6062480718111345e-06}, {0.001131603875, "Field Reading"=4.520781952921487e-06}, {0.0011331272900000002, "Field Reading"=4.494773586767835e-06}, {0.0011473131359999995, "Field Reading"=4.61137276449738e-06}, {0.0011562967579999998, "Field Reading"=4.502464276403611e-06}, {0.0011635118540000002, "Field Reading"=4.4094022313729476e-06}, {0.0011762460965, "Field Reading"=4.598939619318294e-06}, {0.0011869967450000001, "Field Reading"=4.43778070158783e-06}, {0.0011986068415, "Field Reading"=4.533166956190153e-06}, {0.0012075267305, "Field Reading"=4.280196888873947e-06}, {0.0012231219875, "Field Reading"=4.5934078035350194e-06}, {0.0012342542800000003, "Field Reading"=4.691794372932624e-06}, {0.0012452850685, "Field Reading"=4.741253404084463e-06}, {0.001249669164, "Field Reading"=4.7684202380208835e-06}, {0.0012656222550000002, "Field Reading"=4.757546704647578e-06}, {0.0012774779504999998, "Field Reading"=5.033473722435874e-06}, {0.0012884761419999999, "Field Reading"=5.371725684648922e-06}, {0.001302274137, "Field Reading"=5.757185524404366e-06}, {0.001315483442, "Field Reading"=5.989150530511689e-06}, {0.001318617824, "Field Reading"=6.189093863181622e-06}, {0.001326896802, "Field Reading"=6.519691458471505e-06}, {0.0013321671650000002, "Field Reading"=6.257151862260228e-06}, {0.0013382595995, "Field Reading"=6.938678094849753e-06}, {0.0013431049475, "Field Reading"=6.506764220557829e-06}, {0.0013513848205, "Field Reading"=6.392892156791413e-06}, {0.0013605541305, "Field Reading"=6.871823095546326e-06}, {0.0013674233569999999, "Field Reading"=7.061815977729447e-06}, {0.001377506577, "Field Reading"=7.166285840091996e-06}, {0.001384626495, "Field Reading"=7.203151054218705e-06}, {0.0013912282004999998, "Field Reading"=7.1443353170205105e-06}, {0.001397389499, "Field Reading"=7.444518646474147e-06}, {0.0014098793685, "Field Reading"=7.37709053241571e-06}, {0.0014143535475, "Field Reading"=7.663026992951427e-06}, {0.0014176051145, "Field Reading"=7.63857179224e-06}, {0.001422531716, "Field Reading"=8.008615196700489e-06}, {0.0014183687095, "Field Reading"=7.895237542278123e-06}, {0.001434766712, "Field Reading"=9.161836798892856e-06}, {0.0014421111175, "Field Reading"=8.57561560600896e-06}, {0.0014465123884999998, "Field Reading"=8.636993936082646e-06}, {0.0014471561780000002, "Field Reading"=8.636026555121246e-06}, {0.0014508354315000002, "Field Reading"=9.340521117844613e-06}, {0.001465194156, "Field Reading"=8.874806378071606e-06}, {0.001471227326, "Field Reading"=9.030583339093065e-06}, {0.0014737817015, "Field Reading"=9.247947335792214e-06}, {0.001477593292, "Field Reading"=9.290622903194133e-06}, {0.0014860504115, "Field Reading"=9.505263105621828e-06}, {0.0014891984095, "Field Reading"=9.34153271035374e-06}, {0.0014939562035000003, "Field Reading"=1.0270367382838764e-05}, {0.0015029994485, "Field Reading"=1.0113637792160576e-05}, {0.0015062711935, "Field Reading"=1.0195656968551517e-05}, {0.0015124728019999998, "Field Reading"=1.0014883839856853e-05}, {0.001519180098, "Field Reading"=1.0328441991132904e-05}, {0.0015278149494999998, "Field Reading"=1.0164421939934186e-05}, {0.0015282128515000002, "Field Reading"=1.026517627580314e-05}, {0.0015261484435, "Field Reading"=1.0442065912807572e-05}, {0.0015370505819999997, "Field Reading"=1.0852299766404222e-05}, {0.0015386003745, "Field Reading"=1.0494077396609419e-05}, {0.0015355722305000002, "Field Reading"=1.1036339960562228e-05}, {0.0015539013479999998, "Field Reading"=1.0695653585020391e-05}, {0.0015527807625, "Field Reading"=1.1168076593077618e-05}, {0.0015487510525, "Field Reading"=1.1548518836017154e-05}, {0.001559612833, "Field Reading"=1.1280389499271756e-05}, {0.0015726171459999997, "Field Reading"=1.1125196288390165e-05}, {0.0015752137195000002, "Field Reading"=1.1700396035561211e-05}, {0.0015787827725, "Field Reading"=1.1560233899737552e-05}, {0.0015863119115, "Field Reading"=1.1499857870966196e-05}, {0.001592644974, "Field Reading"=1.1799810023087886e-05}, {0.0015930805365000002, "Field Reading"=1.1909281968019716e-05}, {0.0015899645494999999, "Field Reading"=1.1998928879703877e-05}, {0.0015817656669999999, "Field Reading"=1.2023652969289561e-05}, {0.0015890378035, "Field Reading"=1.1966408093048177e-05}, {0.0015987924094999998, "Field Reading"=1.2038736015966978e-05}, {0.0015975906790000002, "Field Reading"=1.196274038933148e-05}, {0.001600574338, "Field Reading"=1.2107982527751793e-05}, {0.0016086013449999998, "Field Reading"=1.2034075080885238e-05}, {0.0016151453515, "Field Reading"=1.2037841981714661e-05}, {0.0016101236585000002, "Field Reading"=1.221645192748754e-05}, {0.0016113429459999999, "Field Reading"=1.2321896914082814e-05}, {0.0016209279949999998, "Field Reading"=1.2222415422845432e-05}, {0.0016241759255000003, "Field Reading"=1.23102694694239e-05}, {0.0016228086995000001, "Field Reading"=1.2256511311411042e-05}, {0.001634366717, "Field Reading"=1.2456860232487586e-05}, {0.0016346827015000002, "Field Reading"=1.2371901884655317e-05}, {0.0016399640375, "Field Reading"=1.2379474136762e-05}, {0.0016437035345, "Field Reading"=1.2497593210412343e-05}, {0.001646538266, "Field Reading"=1.2602051376017006e-05}, {0.0016512208145000001, "Field Reading"=1.2672235147790015e-05}, {0.0016499661754999998, "Field Reading"=1.246246156435146e-05}, {0.0016553584010000001, "Field Reading"=1.2468470696765571e-05}, {0.0016657569905, "Field Reading"=1.2712357440819713e-05}, {0.0016710401725000001, "Field Reading"=1.2694627790432736e-05}, {0.0016728186465, "Field Reading"=1.2406108154483099e-05}, {0.0016732655669999996, "Field Reading"=1.2442856033763291e-05}, {0.0016827645545, "Field Reading"=1.2644716984839226e-05}, {0.001685907737, "Field Reading"=1.2614479932664251e-05}, {0.001682973122, "Field Reading"=1.3028631031311927e-05}, {0.0016979141035000003, "Field Reading"=1.2606663784092668e-05}, {0.001698071667, "Field Reading"=1.2783598025724303e-05}, {0.0017044130895, "Field Reading"=1.2690257237821475e-05}, {0.0017034586310000002, "Field Reading"=1.2721486177144678e-05}, {0.0017042625860000005, "Field Reading"=1.2496261118269682e-05}, {0.0017199405964999997, "Field Reading"=1.3490953434209594e-05}, {0.0017254024279999998, "Field Reading"=1.3534639608853072e-05}, {0.001727302312, "Field Reading"=1.3491335033099144e-05}, {0.0017392099649999999, "Field Reading"=1.3951385397514887e-05}, {0.001735487238, "Field Reading"=1.370359647776324e-05}, {0.0017374940865, "Field Reading"=1.3581146255985215e-05}, {0.0017398523484999998, "Field Reading"=1.3930107353657362e-05}, {0.0017450798240000003, "Field Reading"=1.4078068631250827e-05}, {0.0017491457834999998, "Field Reading"=1.3921280320993627e-05}, {0.0017501297199999997, "Field Reading"=1.414255536369368e-05}, {0.0017569741669999999, "Field Reading"=1.401114336621889e-05}, {0.0017535224749999998, "Field Reading"=1.3946941897587539e-05}, {0.0017618102179999997, "Field Reading"=1.4208882064328718e-05}, {0.0017670795415, "Field Reading"=1.398129461682999e-05}, {0.0017734628075000004, "Field Reading"=1.4109296120679447e-05}, {0.0017746736744999997, "Field Reading"=1.4389352747917243e-05}, {0.0017788715939999998, "Field Reading"=1.2867904761744768e-05}, {0.0017804483450000006, "Field Reading"=1.2944980714226593e-05}, {0.0017815391279999999, "Field Reading"=1.307595550068042e-05}, {0.0017815391730000001, "Field Reading"=1.290657300664517e-05}, {0.001795763225, "Field Reading"=1.3105297968797101e-05}, {0.0017904642679999999, "Field Reading"=1.3074266133083621e-05}, {0.0017996218049999998, "Field Reading"=1.3162573167641184e-05}, {0.0018046273505000002, "Field Reading"=1.3224181246976953e-05}, {0.0018146380275000003, "Field Reading"=1.2931384344000118e-05}, {0.0018158670905, "Field Reading"=1.2894787362623312e-05}, {0.0018113002495000002, "Field Reading"=1.2968656669974477e-05}, {0.0018172502940000002, "Field Reading"=1.3422061982036909e-05}, {0.0018203601454999997, "Field Reading"=1.3798972312619975e-05}, {0.0018257998594999997, "Field Reading"=1.3817025726477106e-05}, {0.0018260027340000003, "Field Reading"=1.3743064521270043e-05}, {0.001829699397, "Field Reading"=1.3504979133192324e-05}, {0.001831783035, "Field Reading"=1.375678535320515e-05}, {0.0018357739915000001, "Field Reading"=1.3351281184093638e-05}, {0.0018411794015000004, "Field Reading"=1.3352889363676527e-05}, {0.0018457646564999995, "Field Reading"=1.3435225712547088e-05}, {0.001850347914, "Field Reading"=1.3453571324902082e-05}, {0.0018517845580000001, "Field Reading"=1.3569482662343788e-05}, {0.0018576741015, "Field Reading"=1.3702147369485664e-05}, {0.0018612731595, "Field Reading"=1.3800188374465495e-05}, {0.0018666439234999999, "Field Reading"=1.3555532260735725e-05}, {0.0018635848909999999, "Field Reading"=1.349455763435799e-05}, {0.0018696842985, "Field Reading"=1.327935473509365e-05}, {0.001876560852, "Field Reading"=1.345953601085484e-05}, {0.001876178283, "Field Reading"=1.360620925087754e-05}, {0.001879944196, "Field Reading"=1.3607664116851746e-05}, {0.0018831122134999995, "Field Reading"=1.3564513025193222e-05}, {0.0018858618519999998, "Field Reading"=1.3466381703392944e-05}, {0.0018929087360000003, "Field Reading"=1.3088879540483008e-05}, {0.001902232718, "Field Reading"=1.3365312280267946e-05}, {0.0019048929500000002, "Field Reading"=1.3585470188750945e-05}, {0.0019029311955000004, "Field Reading"=1.3360654811247516e-05}, {0.0019113146650000003, "Field Reading"=1.3381370117743072e-05}, {0.001914038602, "Field Reading"=1.3237107856925436e-05}, {0.0019139526260000001, "Field Reading"=1.353940866861469e-05}, {0.0019203413650000002, "Field Reading"=1.3324462926848481e-05}, {0.001929312534, "Field Reading"=1.3439688188057686e-05}, {0.0019328294555000004, "Field Reading"=1.3434948409426759e-05}, {0.0019311340364999998, "Field Reading"=1.3306206206422427e-05}, {0.0019388599010000001, "Field Reading"=1.3436539903912318e-05}, {0.0019388791899999998, "Field Reading"=1.3185696935704067e-05}, {0.001940390082, "Field Reading"=1.3365845517215295e-05}, {0.0019443058230000005, "Field Reading"=1.3200286194010101e-05}, {0.0019463944060000003, "Field Reading"=1.3389918686264318e-05}, {0.0019495602859999999, "Field Reading"=1.3426043969596405e-05}, {0.001957699042, "Field Reading"=1.3259038749775481e-05}, {0.0019599970525000002, "Field Reading"=1.3370749359056993e-05}, {0.001964974775, "Field Reading"=1.3226760659915391e-05}, {0.001971763734, "Field Reading"=1.3348397714547647e-05}, {0.0019709724890000003, "Field Reading"=1.3213097047834592e-05}, {0.001973912851, "Field Reading"=1.2927563187976859e-05}, {0.0019786452289999997, "Field Reading"=1.3381691998478692e-05}, {0.0019861288344999997, "Field Reading"=1.3294535143953758e-05}, {0.0019905205964999995, "Field Reading"=1.3198661457188184e-05}, {0.0019891819465, "Field Reading"=1.3226422732138774e-05}, {0.0019983655345, "Field Reading"=1.3219364846342082e-05}, {0.002001699916, "Field Reading"=1.3135170937012063e-05}, {0.0020040525959999994, "Field Reading"=1.324011558429505e-05}, {0.0020080957920000004, "Field Reading"=1.3014121476663512e-05}, {0.0020122820280000005, "Field Reading"=1.3360084699751845e-05}, {0.002017432494, "Field Reading"=1.3189988642690668e-05}, {0.0020232491795000003, "Field Reading"=1.3153667793690079e-05}, {0.0020239178795000002, "Field Reading"=1.3171322833396517e-05}, {0.0020281289575000004, "Field Reading"=1.3376768308345061e-05}, {0.002032242117, "Field Reading"=1.3086822415273864e-05}, {0.0020366120495, "Field Reading"=1.3163712830656927e-05}, {0.002037284367, "Field Reading"=1.3228618236141174e-05}, {0.0020424433815, "Field Reading"=1.3042001000659411e-05}, {0.0020505932470000006, "Field Reading"=1.298242218608853e-05}, {0.0020523757095, "Field Reading"=1.3131833211481508e-05}, {0.0020552329075, "Field Reading"=1.3164183468047156e-05}, {0.0020582330124999998, "Field Reading"=1.314001232437387e-05}, {0.0020602470605, "Field Reading"=1.2984706464374603e-05}, {0.002066759857, "Field Reading"=1.304270452576241e-05}, {0.0020698684505, "Field Reading"=1.343512503257213e-05}, {0.0020731791065000003, "Field Reading"=1.322078826614707e-05}, {0.002076803308, "Field Reading"=1.3363905088959904e-05}, {0.0020784948404999996, "Field Reading"=1.33482159898699e-05}, {0.002083340171, "Field Reading"=1.3459948237225242e-05}, {0.0020826984965, "Field Reading"=1.3451780950422405e-05}, {0.0020852244485000003, "Field Reading"=1.3435746410828313e-05}, {0.002088538939, "Field Reading"=1.328160468927274e-05}, {0.0020943668150000005, "Field Reading"=1.3378066720075018e-05}, {0.0020952348440000006, "Field Reading"=1.3298585278437808e-05}, {0.0021000441945, "Field Reading"=1.3354401695395779e-05}, {0.0021043080265, "Field Reading"=1.3168451862298553e-05}, {0.002106308513, "Field Reading"=1.348056330939173e-05}, {0.00210586206, "Field Reading"=1.3158821454062163e-05}, {0.0021138913890000003, "Field Reading"=1.3143563478394125e-05}, {0.0021184450560000003, "Field Reading"=1.3282865810077578e-05}, {0.002125551054, "Field Reading"=1.3237786955585475e-05}, {0.0021247365405, "Field Reading"=1.3145626163680577e-05}, {0.002128095854, "Field Reading"=1.3159699071227118e-05}, {0.0021334296365, "Field Reading"=1.3212379286225272e-05}, {0.0021362148275000004, "Field Reading"=1.3135763142629036e-05}, {0.00214161833, "Field Reading"=1.331152793636621e-05}, {0.0021442808204999997, "Field Reading"=1.3225722276350033e-05}, {0.0021489080329999996, "Field Reading"=1.337279007513106e-05}, {0.0021521562805, "Field Reading"=1.3219231302332895e-05}, {0.0021569279615, "Field Reading"=1.3103740689784974e-05}, {0.002159247329, "Field Reading"=1.3274906077355532e-05}, {0.002166533902, "Field Reading"=1.3466551465156707e-05}, {0.002164887186, "Field Reading"=1.3338144941961428e-05}, {0.0021694527004999997, "Field Reading"=1.3281959456314454e-05}, {0.0021723408064999996, "Field Reading"=1.3378824644708832e-05}, {0.0021790509915, "Field Reading"=1.3359241160811905e-05}, {0.0021858921884999995, "Field Reading"=1.3457152212095877e-05}, {0.0021909930865, "Field Reading"=1.3285506109486149e-05}, {0.0021932943759999995, "Field Reading"=1.3745923281126733e-05}, {0.0021994255709999995, "Field Reading"=1.3377631199503405e-05}, {0.002204951217, "Field Reading"=1.3417062681697916e-05}, {0.0022081393995000004, "Field Reading"=1.344705283631882e-05}, {0.002211472162, "Field Reading"=1.3394398453572953e-05}, {0.0022177148285, "Field Reading"=1.3507305057908734e-05}, {0.0022191600595, "Field Reading"=1.3402011990115535e-05}, {0.0022230627625, "Field Reading"=1.3462393824349452e-05}, {0.0022272719285, "Field Reading"=1.3444598357128956e-05}, {0.0022315120465, "Field Reading"=1.3485838290656972e-05}, {0.002235793674, "Field Reading"=1.3526717025421753e-05}, {0.0022410807954999995, "Field Reading"=1.3486132257912043e-05}, {0.0022429617550000004, "Field Reading"=1.3434121568275324e-05}, {0.0022493792475, "Field Reading"=1.3189456767490661e-05}, {0.0022530698465, "Field Reading"=1.3457475466107694e-05}, {0.0022519914835, "Field Reading"=1.3517350393505597e-05}, {0.0022524006135, "Field Reading"=1.3600814225670048e-05}, {0.0022578569765000006, "Field Reading"=1.3503598716857563e-05}, {0.0022583190265000005, "Field Reading"=1.3448789022732667e-05}, {0.0022633971439999997, "Field Reading"=1.34597885607888e-05}, {0.0022664268640000002, "Field Reading"=1.3639079102196108e-05}, {0.0022708191659999996, "Field Reading"=1.3762023848052756e-05}, {0.0022751014755, "Field Reading"=1.3545563789227516e-05}, {0.0022739796009999995, "Field Reading"=1.3514982582232331e-05}, {0.0022788035189999995, "Field Reading"=1.3431281384278807e-05}, {0.0022806122224999998, "Field Reading"=1.3483712180033955e-05}, {0.0022852916425000003, "Field Reading"=1.3442076285047663e-05}, {0.002292193286, "Field Reading"=1.3515728472776278e-05}, {0.0022958791484999994, "Field Reading"=1.3593553624673628e-05}, {0.0023032794395, "Field Reading"=1.355145012918507e-05}, {0.0023059863195, "Field Reading"=1.3314972951368184e-05}, {0.0023050398475, "Field Reading"=1.3599920772376534e-05}, {0.0023106814414999995, "Field Reading"=1.3395813474347817e-05}, {0.002316534312, "Field Reading"=1.3607973193703977e-05}, {0.002319406965, "Field Reading"=1.3600031659108832e-05}, {0.0023283312060000004, "Field Reading"=1.3406239348745139e-05}, {0.0023307445805, "Field Reading"=1.3538164624209587e-05}, {0.00233209636, "Field Reading"=1.3817652724678178e-05}, {0.0023336578535, "Field Reading"=1.348044615446931e-05}, {0.002339671677, "Field Reading"=1.3583317426458159e-05}, {0.0023417782724999997, "Field Reading"=1.3529870233638999e-05}, {0.0023488792919999996, "Field Reading"=1.3546705308555562e-05}, {0.0023514640845, "Field Reading"=1.358498318283932e-05}, {0.0023592918710000003, "Field Reading"=1.3448321575890347e-05}, {0.0023599502340000003, "Field Reading"=1.351454227124961e-05}, {0.002366855691, "Field Reading"=1.3684836480179771e-05}, {0.0023702501305, "Field Reading"=1.3550314614250504e-05}, {0.0023726493889999994, "Field Reading"=1.3444640583655023e-05}, {0.0023792215645, "Field Reading"=1.3599967279876342e-05}, {0.0023822989825000003, "Field Reading"=1.3534790077291047e-05}, {0.0023870874705000005, "Field Reading"=1.354734442372477e-05}, {0.0023899540424999997, "Field Reading"=1.3601583402661505e-05}, {0.0023898244359999996, "Field Reading"=1.355346009792413e-05}, {0.002393079496, "Field Reading"=1.335095120468286e-05}, {0.0023994568800000003, "Field Reading"=1.3654746908645311e-05}, {0.002399925307, "Field Reading"=1.3543174757426775e-05}, {0.002403106708, "Field Reading"=1.367767029995066e-05}, {0.002404012533, "Field Reading"=1.3476350337100556e-05}, {0.0024075422669999997, "Field Reading"=1.3501841098117499e-05}, {0.0024142210889999995, "Field Reading"=1.3526689561348296e-05}, {0.002418345375, "Field Reading"=1.347289187207651e-05}, {0.0024137838819999996, "Field Reading"=1.3630495922165079e-05}, {0.0024181997905000007, "Field Reading"=1.3582224457345251e-05}]
  out "data":dbl[](array[numeric])=[-3.778e-06, 17571.544, 0.0024181997905000007, 2.300252839072771e-10, 1.6935759280791425e-05, 1.3582224457345251e-05, -1.5999999999999879, -7.999999999999939e-08]
  in  "Nanovoltmeter 2182a VISA":refnum<visa-resource-name>="GPIB0::4::INSTR"
  in  "Step":dbl[](array[numeric])=[0.0005] min=-3000.0 max=3000.0 format="%.1e"
  in  "To":dbl[](array[numeric])=[-0.06] min=-3000.0 max=3000.0 format="%.1e"
  in  "From":dbl[](array[numeric])=[0.06] min=-3000.0 max=3000.0 format="%.1e"
  in  "file name":string="007_MA2678_[Dev50]_dI-dV(H)_12uV_970pA_17.7777Hz_4thorder_300ms_0T_measureR_20xaverage"
  out "File path":path=path "D:/Pranava/Data/STS/MA2087/025_MA2087_STS_[Dev100]_baseT_0T_37uV_137.919Hz_float_100xaverage.dat"
  # ".dat"
  # "Set Voltage (V)"
  # "Set Magnetic Field (T)"
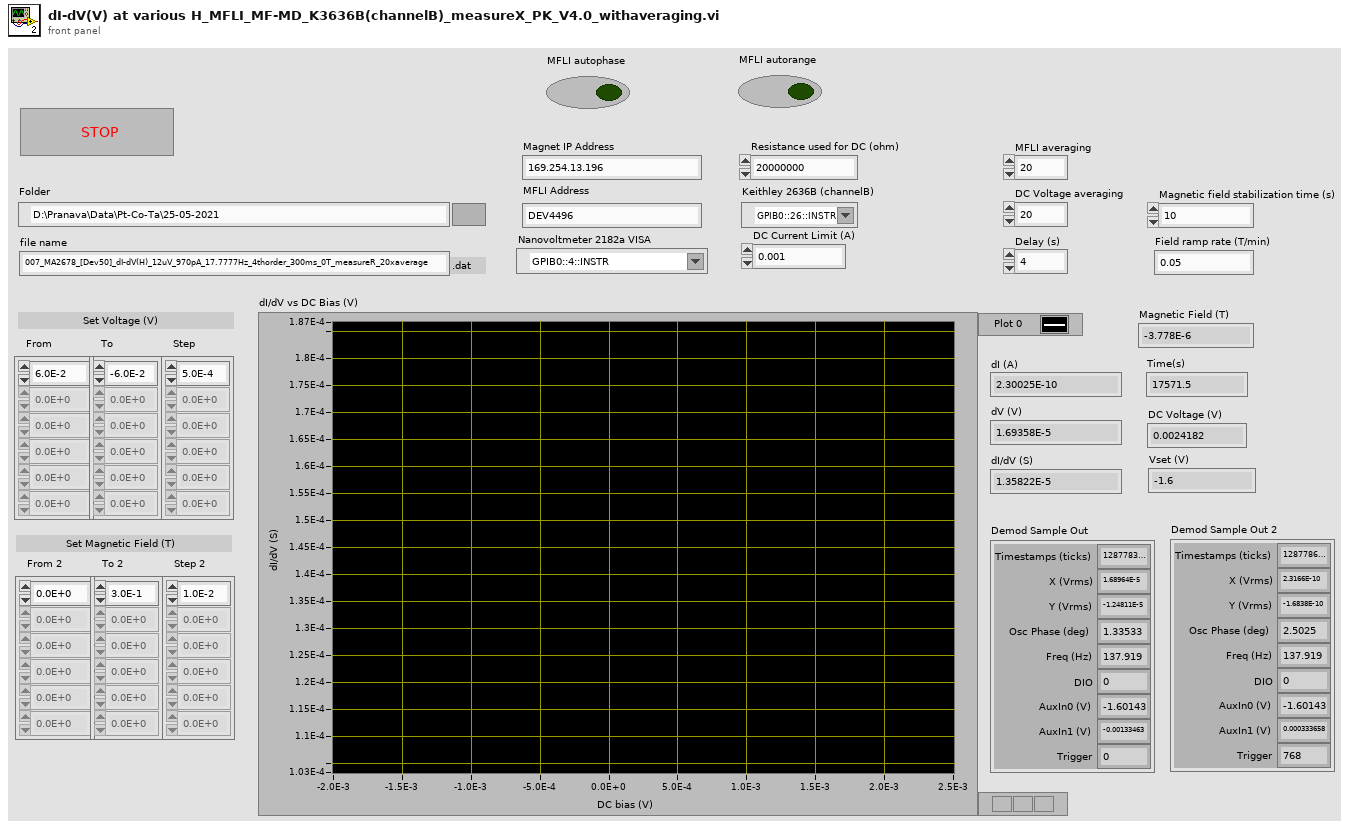
[diagram p1: front panel]
types:
  T1 = typedef "Zurich Instruments LabOne.lvlib/ziTypeDemodSampleSingle.ctl" = cluster{"Timestamps (ticks)":u64, "X (Vrms)":dbl, "Y (Vrms)":dbl, "Osc Phase (deg)":dbl, "Freq (Hz)":dbl, "DIO":u32, "AuxIn0 (V)":dbl, "AuxIn1 (V)":dbl, "Trigger":u32}
  T2 = enum16{"open", "replace", "create", "open or create", "replace or create", "replace or create with confirmation"}
  T3 = typedef "Zurich Instruments LabOne.lvlib/ziTypeHandle.ctl" = cluster{"handleValid":bool, "Conn":u64, "Path Prefix":string, "Handle":u64, "Connected":bool, "Clockbase(s)":dbl}
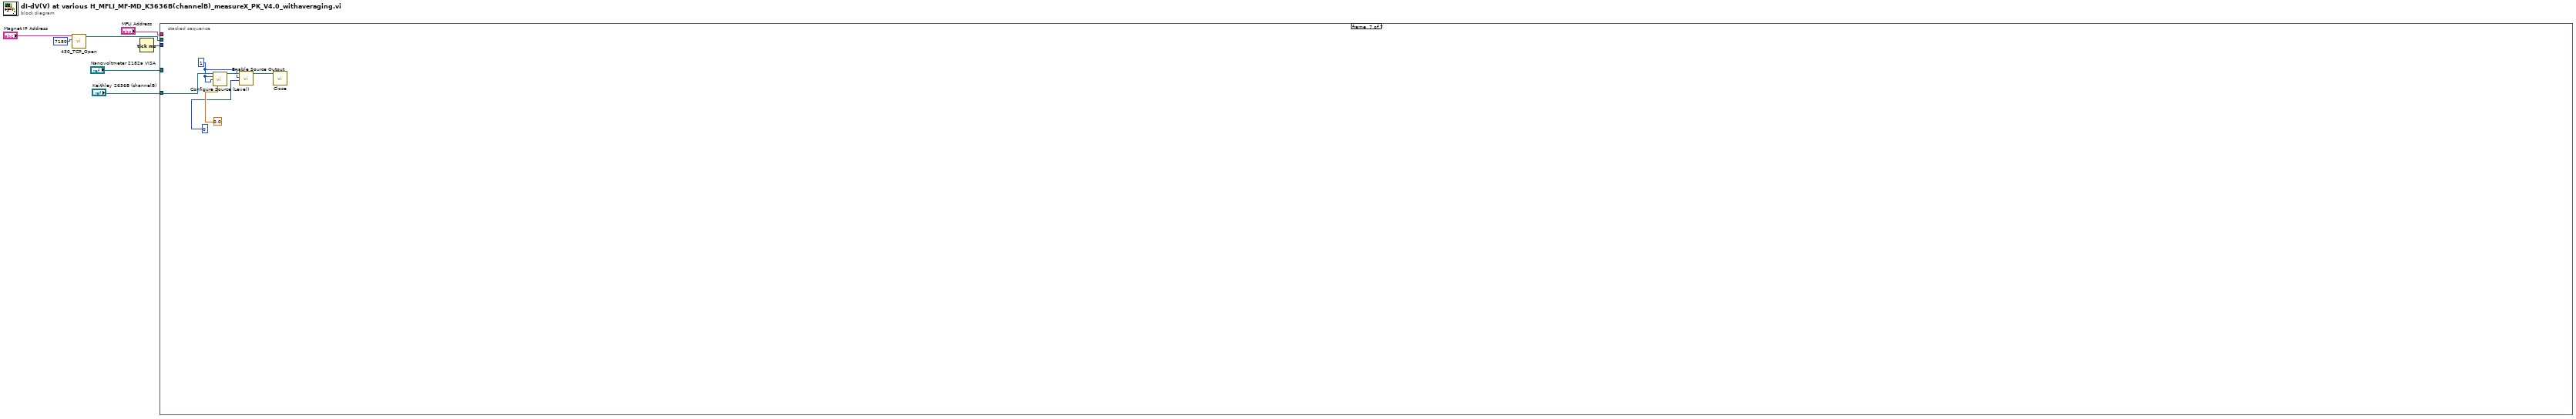
[diagram p0: block diagram]
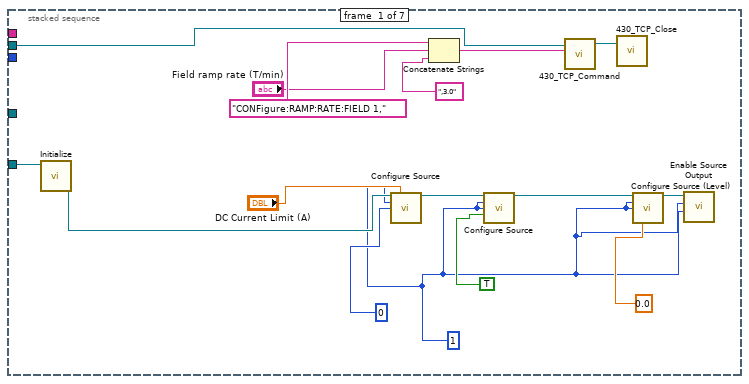
[diagram p2: hidden frame]
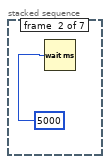
[diagram p3: hidden frame]
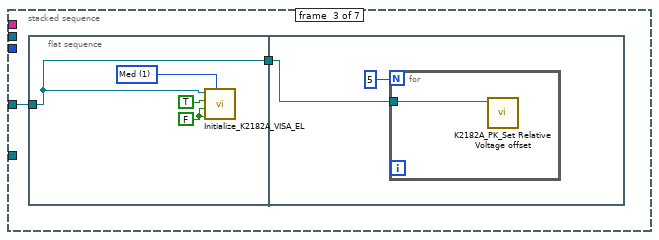
[diagram p4: hidden frame]
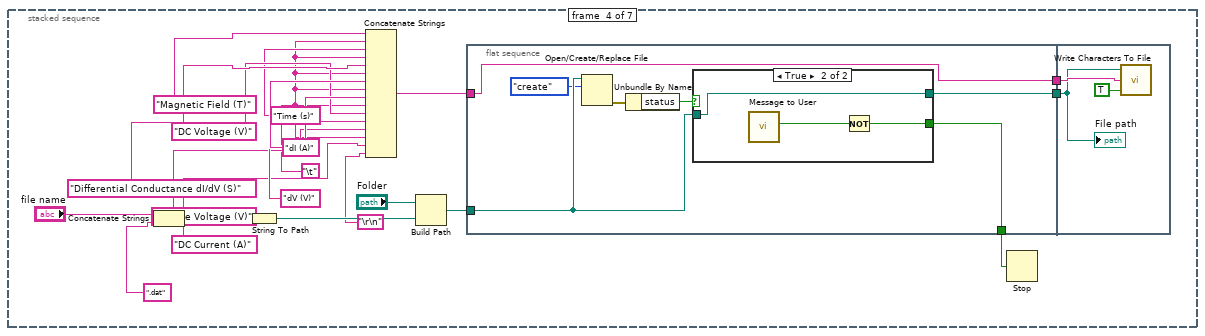
[diagram p5: hidden frame]
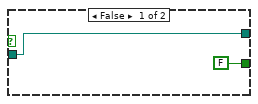
[diagram p6: hidden frame]
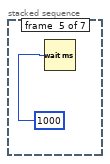
[diagram p7: hidden frame]
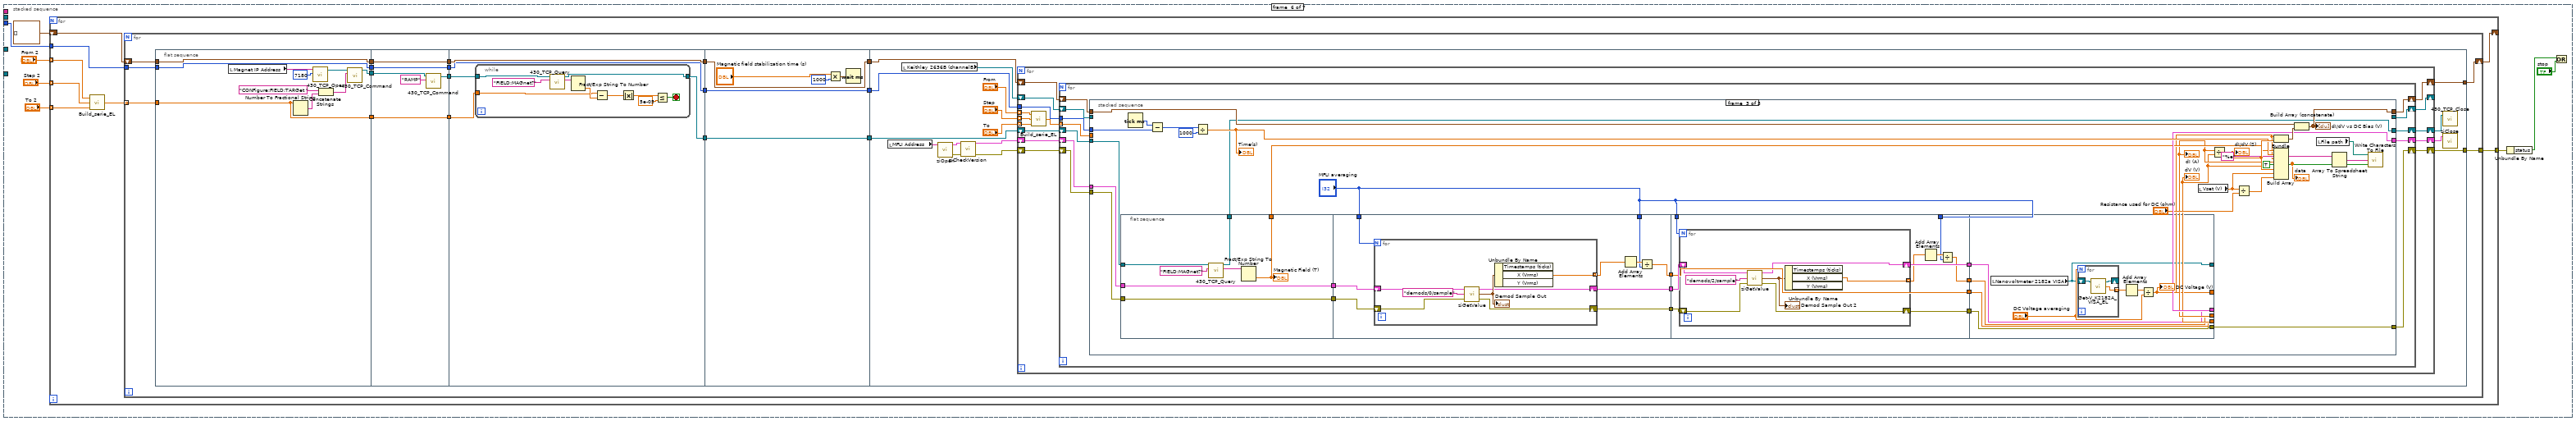
[diagram p8: hidden frame]
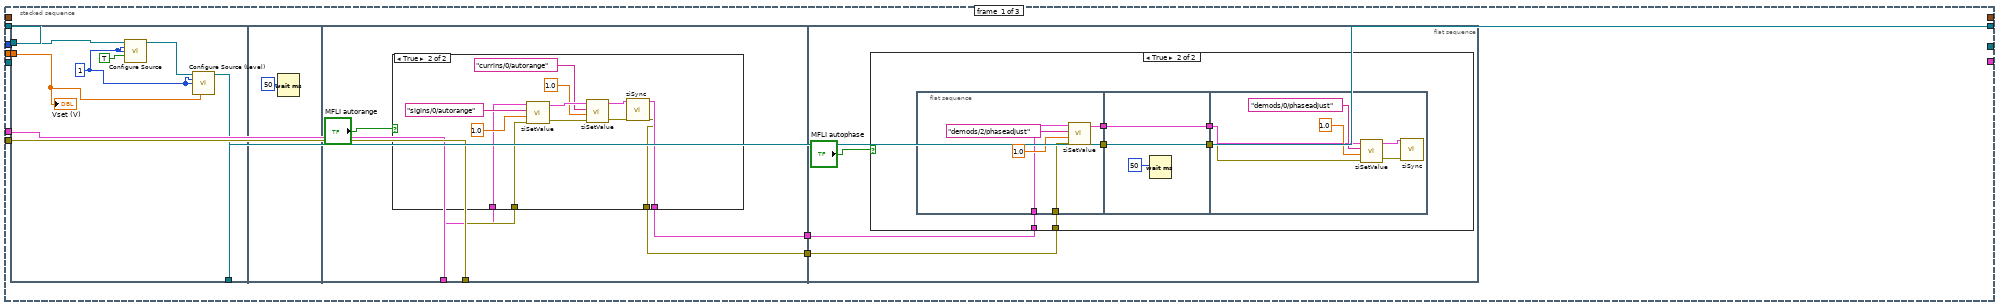
[diagram p9: hidden frame]
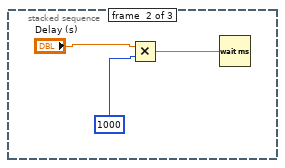
[diagram p12: hidden frame]
diagram:
  n1 = call "430_TCP_Open.vi"("IP Address"="Magnet IP Address", "TCP Port"=7180) -> ("connection ID"=w2:refnum<k5>)  [unwired: 4 in, 2 out]
  n2 = Tick Count (ms)() -> (millisecond timer value=w5:u32)
  n3 = stacked-sequence {
    tunnel: "Nanovoltmeter 2182a VISA" -> [_ _ w26 _ _ _ _]
    tunnel: "MFLI Address" -> [_ _ _ _ _ _ _]
    tunnel: w5 -> [_ _ _ _ _ w76 _]
    tunnel: w2 -> [w18 _ _ _ _ _ _]
    tunnel: "Keithley 2636B (channelB)" -> [w17 _ _ _ _ _ w335]
    frame #0 {
      w8 = 1
      n4 = call <instrlib>:"Initialize.vi"("VISA resource name"=w17) -> ("VISA resource name out"=w16:refnum<visa-resource-name>)  [unwired: 9 in, 1 out]
      n5 = call-poly <instrlib>:"Configure Source.vi"("VISA resource name"=w16, "Current Limit (0.1 A)"="DC Current Limit (A)", "Source Measure Unit Channel (0: Channel A)"=w8, "Limit Type (1: Voltage)"=0) -> ("VISA resource name out"=w15:refnum<visa-resource-name>)  [unwired: 10 in, 1 out]
      n6 = Concatenate Strings("CONFigure:RAMP:RATE:FIELD 1," ("String"), "Field ramp rate (T/min)", ",3.0") -> (w19:string)
      n7 = call-poly <instrlib>:"Configure Source.vi"("VISA resource name"=w15, "Source Measure Unit Channel (0: Channel A)"=w8, "Range Type (1: Voltage)"=w8, "Auto Range (T: Enable)"=TRUE) -> ("VISA resource name out"=w14:refnum<visa-resource-name>)  [unwired: 10 in, 1 out]
      n8 = call "430_TCP_Command.vi"("Command"=w19, "connection ID"=w18) -> ("connection ID out"=w23:refnum<k5>)  [unwired: 2 in, 2 out]
      n9 = call "430_TCP_Close.vi"("connection ID"=w23) -> ()  [unwired: 1 in, 2 out]
      n10 = call <instrlib>:"Configure Source (Level).vi"("VISA resource name"=w14, "Source Measure Unit Channel (0: Channel A)"=w8, "Level Type (1: Voltage)"=w8, "Voltage Level (0 V)"=0.0) -> ("VISA resource name out"=w13:refnum<visa-resource-name>)  [unwired: 10 in, 1 out]
      n11 = call <instrlib>:"Enable Source Output.vi"("Output Mode (0: Turn off)"=w8, "Source Measure Unit Channel (0: Channel A)"=w8, "VISA resource name"=w13) -> ()  [unwired: 7 in, 2 out]
    }
    frame #1 {
      n12 = Wait (ms)(milliseconds to wait=5000) -> ()  [unwired: 1 out]
    }
    frame #2 {
      n13 = flat-sequence {
        tunnel: w26 -> [w27]
        tunnel: [w27] -> w25
        tunnel: w25 -> [w31]
        frame #0 {
          w29 = u16 1 items=["Slow", "Med", "Fast"] ("Rate (NPLC)")
          w30 = FALSE ("Auto range?")
          n14 = call "Initialize_K2182A_VISA_EL.vi"("VISA address"=w27, "Auto range?"=TRUE, "Analog LPass\nFilter?"=w30, "DC\nFilter?"=w30, "Rate (NPLC)"=w29) -> ()  [unwired: 1 in, 1 out]
        }
        frame #1 {
          n15 = for {
            N: 5 ("Numeric") -> [_]
            tunnel: w31 -> [w33]
            n16 = call "K2182A_PK_Set Relative Voltage offset.vi"("VISA address"=w33) -> ()  [unwired: 11 in]
          }
        }
      }
    }
    frame #3 {
      w35 = "\t"
      n17 = Concatenate Strings("file name", ".dat" ("string")) -> (w50:string)
      n18 = String To Path(string=w50) -> (path=w42:path)
      n19 = Concatenate Strings("Magnetic Field (T)", w35, "Time (s)", w35, "DC Voltage (V)" ("string"), w35, "dI (A)" ("string"), w35, "dV (V)" ("string"), w35, "Differential Conductance dI/dV (S)", w35, "Source Voltage (V)", w35, "DC Current (A)", "\r\n") -> (w51:string)
      n20 = Build Path(base path="Folder", name or relative path=w42) -> (appended path=w41:path)
      n21 = flat-sequence {
        tunnel: w41 -> [w57]
        tunnel: w51 -> [w60]
        tunnel: [w60] -> w53
        tunnel: [w59] -> w48
        tunnel: [w58] -> w52
        tunnel: w53 -> [w67]
        tunnel: w52 -> [w66]
        frame #0 {
          n22 = Open/Create/Replace File(file path (use dialog)=w57, operation (0:open)=T2."create") -> (error out=w56:errorcluster)  [unwired: 4 in, 2 out]
          n23 = Unbundle By Name(w56) -> ("status"=w54:bool)
          n24 = case shown="True" w54 {
            tunnel: [FALSE ("Yes") w64] -> w59
            tunnel: [w61 w63] -> w58
            tunnel: w57 -> [w61 w63]
            frame False {
            }
            frame True {
              n25 = call "Message to User"() -> ("Yes"=w65:bool)  [unwired: 10 in, 1 out]
              n26 = Not(x=w65) -> (.not. x?=w64:bool)
            }
          }
        }
        frame #1 {
          n27 = call <vilib>:"Write Characters To File.vi"("append to file? (new file:F)"=TRUE, "character string"=w67, "file path (dialog if empty)"=w66) -> ()  [unwired: 2 in, 1 out]
          "File path" <- w66
        }
      }
      n28 = Stop(stop? (T)=w48) -> ()
    }
    frame #4 {
      n29 = Wait (ms)(milliseconds to wait=u32 1000) -> ()  [unwired: 1 out]
    }
    frame #5 {
      n30 = for {
        tunnel: w76 -> [w84]
        tunnel: "From 2" -> [w83] mode=indexing
        tunnel: "Step 2" -> [w82] mode=indexing
        tunnel: "To 2" -> [w81] mode=indexing
        shift-right: [w80] -> _
        shift-left: cluster{dbl, "Field Reading":dbl}[] [] -> [w85]
        tunnel: [w78] -> w71
        n31 = call "Build_serie_EL.vi"("end value"=w81, "increment"=w82, "start value"=w83) -> ("output array"=w79:dbl[])
        n32 = for {
          tunnel: w84 -> [w95]
          shift-right: [w94] -> w80
          shift-left: w85 -> [w96]
          tunnel: w79 -> [w93] mode=indexing
          tunnel: [w86] -> w78
          n33 = flat-sequence {
            tunnel: w95 -> [w113]
            tunnel: w96 -> [w114]
            tunnel: [w114] -> w104
            tunnel: [w113] -> w103
            tunnel: w93 -> [w105]
            tunnel: [w106] -> w92
            tunnel: [w105] -> w89
            tunnel: [w120] -> w102
            tunnel: [w119] -> w101
            tunnel: w104 -> [w120]
            tunnel: w103 -> [w119]
            tunnel: w92 -> [w117]
            tunnel: [w116] -> w91
            tunnel: [w115] -> w90
            tunnel: w89 -> [w115]
            tunnel: [w125] -> w100
            tunnel: [w124] -> w99
            tunnel: w102 -> [w125]
            tunnel: w101 -> [w124]
            tunnel: w91 -> [w123]
            tunnel: w90 -> [w122]
            tunnel: [w121] -> w87
            tunnel: [w141] -> w98
            tunnel: [w140] -> w97
            tunnel: w100 -> [w141]
            tunnel: w99 -> [w140]
            tunnel: [w136] -> w88
            tunnel: w87 -> [w136]
            tunnel: [w152] -> w86
            tunnel: w98 -> [w154]
            tunnel: w97 -> [w153]
            tunnel: [w151] -> w94
            tunnel: w88 -> [w150]
            frame #0 {
              n34 = local read "Magnet IP Address"() -> (w108:string)
              n35 = Number To Fractional String(number=w105) -> (F-format string=w110:string)  [unwired: 3 in]
              n36 = call "430_TCP_Open.vi"("IP Address"=w108, "TCP Port"=7180) -> ("connection ID"=w107:refnum<k5>)  [unwired: 4 in, 2 out]
              n37 = Concatenate Strings("CONFigure:FIELD:TARGet " ("String"), w110) -> (w112:string)
              n38 = call "430_TCP_Command.vi"("Command"=w112, "connection ID"=w107) -> ("connection ID out"=w106:refnum<k5>)  [unwired: 2 in, 2 out]
            }
            frame #1 {
              n39 = call "430_TCP_Command.vi"("Command"="RAMP", "connection ID"=w117) -> ("connection ID out"=w116:refnum<k5>)  [unwired: 2 in, 2 out]
            }
            frame #2 {
              n40 = while {
                tunnel: w123 -> [w135]
                tunnel: w122 -> [w130]
                tunnel: [w126] -> w121
                stop <- w128 stop-if-true
                n41 = call "430_TCP_Query.vi"("Command"="FIELD:MAGnet?" ("String"), "connection ID"=w135) -> ("Response"=w134:string, "connection ID out"=w126:refnum<k5>)  [unwired: 5 in, 3 out]
                n42 = Fract/Exp String To Number(string=w134) -> (number=w131:dbl)  [unwired: 3 in, 1 out]
                n43 = Subtract(x=w130, y=w131) -> (x-y=w133:dbl)
                n44 = Absolute Value(x=w133) -> (abs(x)=w132:dbl)
                n45 = Less Or Equal?(x=w132, y=5e-05) -> (x <= y?=w128:bool)
              }
            }
            frame #3 {
              n46 = Multiply(x="Magnetic field stabilization time (s)", y=1000) -> (x*y=w138:dbl)
              n47 = Wait (ms)(milliseconds to wait=w138) -> ()  [unwired: 1 out]
            }
            frame #4 {
              n48 = local read "MFLI Address"() -> (w147:string)
              n49 = local read "Keithley 2636B (channelB)"() -> (w142:refnum<visa-resource-name>)
              n50 = call <instrlib>:"ziOpen.vi"("Address"=w147) -> ("Error Out"=w146:errorcluster, "HandleOut"=w149:T3)  [unwired: 3 in, 1 out]
              n51 = call <instrlib>:"ziCheckVersion.vi"("Handle In"=w149, "Error In"=w146) -> ("Handle Out"=w148:T3, "Error Out"=w145:errorcluster)  [unwired: 11 in, 1 out]
              n52 = for {
                tunnel: "From" -> [w169] mode=indexing
                tunnel: "To" -> [w168] mode=indexing
                tunnel: "Step" -> [w167] mode=indexing
                shift-right: [w171] -> w151
                shift-left: w154 -> [w172]
                tunnel: w153 -> [w166]
                shift-right: [w164] -> w144
                shift-left: w148 -> [w165]
                shift-right: [w163] -> w152
                shift-left: w145 -> [w162]
                shift-right: [w160] -> w143
                shift-left: w150 -> [w161]
                shift-right: [w158] -> _
                shift-left: w142 -> [w159]
                n53 = call "Build_serie_EL.vi"("end value"=w168, "increment"=w167, "start value"=w169) -> ("output array"=w170:dbl[])
                n54 = for {
                  tunnel: w170 -> [w184] mode=indexing
                  shift-right: [w182] -> w171
                  shift-left: w172 -> [w183]
                  tunnel: w166 -> [w181]
                  shift-right: [w179] -> w164
                  shift-left: w165 -> [w180]
                  shift-right: [w178] -> w163
                  shift-left: w162 -> [w177]
                  shift-right: [w175] -> w160
                  shift-left: w161 -> [w176]
                  shift-right: [w173] -> w158
                  shift-left: w159 -> [w174]
                  n55 = stacked-sequence {
                    tunnel: w183 -> [_ _ w278]
                    tunnel: w184 -> [w191 _ _]
                    tunnel: [_ _ w277] -> w182
                    tunnel: w181 -> [_ _ w274]
                    tunnel: w180 -> [w187 _ w270]
                    tunnel: [_ _ w269] -> w179
                    tunnel: [_ _ w268] -> w178
                    tunnel: w177 -> [w188 _ w267]
                    tunnel: w176 -> [_ _ w252]
                    tunnel: [_ _ w251] -> w175
                    tunnel: w174 -> [w189 _ _]
                    tunnel: [w190 _ _] -> w173
                    frame #0 {
                      n56 = flat-sequence {
                        tunnel: w191 -> [w197]
                        tunnel: [w196] -> w190
                        tunnel: w189 -> [w195]
                        tunnel: w188 -> [w203]
                        tunnel: w187 -> [w202]
                        tunnel: [w200] -> w186
                        tunnel: [w199] -> w185
                        tunnel: w186 -> [w217]
                        tunnel: w185 -> [w216]
                        frame #0 {
                          w192 = 1
                          n57 = call-poly <instrlib>:"Configure Source.vi"("VISA resource name"=w195, "Source Measure Unit Channel (0: Channel A)"=w192, "Range Type (1: Voltage)"=w192, "Auto Range (T: Enable)"=TRUE) -> ("VISA resource name out"=w193:refnum<visa-resource-name>)  [unwired: 10 in, 1 out]
                          n58 = call <instrlib>:"Configure Source (Level).vi"("VISA resource name"=w193, "Source Measure Unit Channel (0: Channel A)"=w192, "Level Type (1: Voltage)"=w192, "Voltage Level (0 V)"=w197) -> ("VISA resource name out"=w196:refnum<visa-resource-name>)  [unwired: 10 in, 1 out]
                          "Vset (V)" <- w197
                        }
                        frame #1 {
                          n59 = Wait (ms)(milliseconds to wait=50) -> ()  [unwired: 1 out]
                        }
                        frame #2 {
                          n60 = case shown="True" "MFLI autorange" {
                            tunnel: w203 -> [_ w207]
                            tunnel: w202 -> [_ w206]
                            tunnel: [_ w205] -> w200
                            tunnel: [_ w204] -> w199
                            frame False {
                            }
                            frame True {
                              n61 = call-poly <instrlib>:"ziSetValue.vi"("Error In"=w207, "Value"=1.0, "Path"="sigins/0/autorange", "Handle In"=w206) -> ("Error Out"=w213:errorcluster, "Handle Out"=w212:T3)  [unwired: 1 in]
                              n62 = call-poly <instrlib>:"ziSetValue.vi"("Error In"=w213, "Value"=1.0, "Path"="currins/0/autorange", "Handle In"=w212) -> ("Error Out"=w215:errorcluster, "Handle Out"=w214:T3)  [unwired: 1 in]
                              n63 = call <instrlib>:"ziSync.vi"("Handle In"=w214, "Error In"=w215) -> ("Handle Out"=w205:T3, "Error Out"=w204:errorcluster)  [unwired: 12 in]
                            }
                          }
                        }
                        frame #3 {
                          n64 = case shown="True" "MFLI autophase" {
                            tunnel: w216 -> [_ w224]
                            tunnel: w217 -> [_ w223]
                            frame False {
                            }
                            frame True {
                              n65 = flat-sequence {
                                tunnel: w224 -> [w226]
                                tunnel: w223 -> [w225]
                                tunnel: [w230] -> w222
                                tunnel: [w229] -> w220
                                tunnel: w222 -> [w233]
                                tunnel: [w233] -> w221
                                tunnel: w220 -> [w232]
                                tunnel: [w232] -> w219
                                tunnel: w221 -> [w234]
                                tunnel: w219 -> [w235]
                                frame #0 {
                                n66 = call-poly <instrlib>:"ziSetValue.vi"("Error In"=w226, "Value"=1.0, "Path"="demods/2/phaseadjust", "Handle In"=w225) -> ("Error Out"=w230:errorcluster, "Handle Out"=w229:T3)  [unwired: 1 in]
                                }
                                frame #1 {
                                n67 = Wait (ms)(milliseconds to wait=50) -> ()  [unwired: 1 out]
                                }
                                frame #2 {
                                n68 = call-poly <instrlib>:"ziSetValue.vi"("Error In"=w234, "Value"=1.0, "Path"="demods/0/phaseadjust", "Handle In"=w235) -> ("Error Out"=w236:errorcluster, "Handle Out"=w237:T3)  [unwired: 1 in]
                                n69 = call <instrlib>:"ziSync.vi"("Handle In"=w237, "Error In"=w236) -> ()  [unwired: 12 in, 2 out]
                                }
                              }
                            }
                          }
                        }
                      }
                    }
                    frame #1 {
                      n70 = Multiply(x="Delay (s)", y=1000) -> (x*y=w241:dbl)
                      n71 = Wait (ms)(milliseconds to wait=w241) -> ()  [unwired: 1 out]
                    }
                    frame #2 {
                      n72 = flat-sequence {
                        tunnel: w267 -> [w285]
                        tunnel: w270 -> [w286]
                        tunnel: [w286] -> w254
                        tunnel: [w285] -> w253
                        tunnel: w252 -> [w282]
                        tunnel: [w281] -> w251
                        tunnel: [w280] -> w250
                        tunnel: [w293] -> w261
                        tunnel: [w292] -> w260
                        tunnel: [w289] -> w259
                        tunnel: w254 -> [w295]
                        tunnel: w253 -> [w294]
                        tunnel: "MFLI averaging" -> [w288]
                        tunnel: "MFLI averaging" -> [w287]
                        tunnel: w261 -> [w312]
                        tunnel: w260 -> [w311]
                        tunnel: w259 -> [w308]
                        tunnel: [w310] -> w258
                        tunnel: [w309] -> w257
                        tunnel: [w306] -> w256
                        tunnel: [w308] -> w255
                        tunnel: "MFLI averaging" -> [w304]
                        tunnel: "MFLI averaging" -> [w303]
                        tunnel: [w325] -> w246
                        tunnel: [w326] -> w247
                        tunnel: [w327] -> w268
                        tunnel: [w328] -> w269
                        tunnel: w258 -> [w328]
                        tunnel: w257 -> [w327]
                        tunnel: w256 -> [w326]
                        tunnel: w255 -> [w325]
                        tunnel: [w322] -> w245
                        tunnel: [w320] -> _
                        frame #0 {
                          n73 = call "430_TCP_Query.vi"("Command"="FIELD:MAGnet?" ("String"), "connection ID"=w282) -> ("Response"=w284:string, "connection ID out"=w281:refnum<k5>)  [unwired: 5 in, 3 out]
                          n74 = Fract/Exp String To Number(string=w284) -> (number=w280:dbl)  [unwired: 3 in, 1 out]
                          "Magnetic Field (T)" <- w280
                        }
                        frame #1 {
                          n75 = for {
                            N: w287 -> [_]
                            tunnel: [w296] -> w290 mode=indexing
                            shift-right: [w298] -> w293
                            shift-left: w295 -> [w300]
                            shift-right: [w297] -> w292
                            shift-left: w294 -> [w299]
                            n76 = call-poly <instrlib>:"ziGetValue.vi"("error in"=w299, "Path"="demods/0/sample", "Handle In"=w300) -> ("error out"=w297:errorcluster, "Demod Sample Out"=w301:T1, "Handle Out"=w298:T3)
                            "Demod Sample Out" <- w301
                            n77 = Unbundle By Name(w301) -> ("X (Vrms)"=w296:dbl)  [unwired: 2 out]
                          }
                          n78 = Add Array Elements(numeric array=w290) -> (sum=w291:dbl)
                          n79 = Divide(x=w291, y=w288) -> (x/y=w289:dbl)
                        }
                        frame #2 {
                          n80 = for {
                            N: w303 -> [_]
                            tunnel: [w313] -> w305 mode=indexing
                            shift-right: [w315] -> w310
                            shift-left: w312 -> [w317]
                            shift-right: [w314] -> w309
                            shift-left: w311 -> [w316]
                            n81 = call-poly <instrlib>:"ziGetValue.vi"("error in"=w316, "Path"="demods/2/sample", "Handle In"=w317) -> ("error out"=w314:errorcluster, "Demod Sample Out"=w318:T1, "Handle Out"=w315:T3)
                            "Demod Sample Out 2" <- w318
                            n82 = Unbundle By Name(w318) -> ("X (Vrms)"=w313:dbl)  [unwired: 2 out]
                          }
                          n83 = Add Array Elements(numeric array=w305) -> (sum=w307:dbl)
                          n84 = Divide(x=w307, y=w304) -> (x/y=w306:dbl)
                        }
                        frame #3 {
                          n85 = local read "Nanovoltmeter 2182a VISA"() -> (w320:refnum<visa-resource-name>)
                          n86 = for {
                            N: "DC Voltage averaging" -> [_]
                            tunnel: [w330] -> w323 mode=indexing
                            shift-right: [w329] -> _
                            shift-left: w320 -> [w331]
                            n87 = call "Get-V_K2182A_VISA_EL.vi"("VISA K2182A"=w331) -> ("V (V)"=w330:dbl, "VISA K2182A"=w329:refnum<visa-resource-name>)  [unwired: 2 in, 1 out]
                          }
                          n88 = Add Array Elements(numeric array=w323) -> (sum=w324:dbl)
                          n89 = Divide(x=w324, y="DC Voltage averaging") -> (x/y=w322:dbl)
                          "DC Voltage (V)" <- w322
                        }
                      }
                      n90 = Tick Count (ms)() -> (millisecond timer value=w275:u32)
                      n91 = Subtract(x=w275, y=w274) -> (x-y=w273:u32)
                      n92 = Divide(x=w273, y=1000) -> (x/y=w271:dbl)
                      "Time(s)" <- w271
                      n93 = local read "Vset (V)"() -> (w248:dbl)
                      n94 = Divide(x=w247, y=w246) -> (x/y=w276:dbl)
                      "dI/dV (S)" <- w276
                      n95 = Divide(x=w248, y="Resistance used for DC (ohm)") -> (x/y=w244:dbl)
                      n96 = Bundle(w245, w276) -> (w279:cluster{dbl, dbl})  [unwired: 1 in]
                      n97 = Build Array(w250, w271, w245, w247, w246, w276, w248, w244) -> (w262:dbl[])
                      "data" <- w262
                      n98 = Build Array (concatenate)(w278, w279) -> (w277:cluster{dbl, "Field Reading":dbl}[])
                      "dI/dV vs DC Bias (V)" <- w277
                      n99 = local read "File path"() -> (w264:path)
                      n100 = Array To Spreadsheet String(array=w262, 3:"%e" ("format string")) -> (spreadsheet string=w265:string)  [unwired: 1 in]
                      n101 = call <vilib>:"Write Characters To File.vi"("append to file? (new file:F)"=TRUE, "character string"=w265, "file path (dialog if empty)"=w264) -> ()  [unwired: 2 in, 1 out]
                      "dI (A)" <- w247
                      "dV (V)" <- w246
                    }
                  }
                }
              }
              n102 = call "430_TCP_Close.vi"("connection ID"=w143) -> ()  [unwired: 1 in, 2 out]
              n103 = call <instrlib>:"ziClose.vi"("Handle In"=w144) -> ()  [unwired: 1 in, 4 out]
            }
          }
        }
      }
      n104 = Unbundle By Name(w71) -> ("status"=w70:bool)
      n105 = Or(x=w70, y="stop") -> ()  [unwired: 1 out]
    }
    frame #6 {
      w332 = 1
      n106 = call <instrlib>:"Configure Source (Level).vi"("VISA resource name"=w335, "Source Measure Unit Channel (0: Channel A)"=w332, "Level Type (1: Voltage)"=w332, "Voltage Level (0 V)"=0.0) -> ("VISA resource name out"=w337:refnum<visa-resource-name>)  [unwired: 10 in, 1 out]
      n107 = call <instrlib>:"Enable Source Output.vi"("Output Mode (0: Turn off)"=0, "Source Measure Unit Channel (0: Channel A)"=w332, "VISA resource name"=w337) -> ("VISA resource name out"=w333:refnum<visa-resource-name>)  [unwired: 7 in, 1 out]
      n108 = call <instrlib>:"Close.vi"("VISA resource name"=w333) -> ()  [unwired: 10 in, 1 out]
    }
  }
